vi "Main Scratch Module.vi"(8 "error in (no error)":errorcluster, 11 "main ref":T1) -> (0 "error out":errorcluster)   [LabVIEW 2025]
uses:
  controls/LAB-IQ UI Data.ctl
  Scratch Main Enum.ctl
  HEAVE vi's/Heave Write enum.ctl
  b016255a-5e45-488d-a19e-9ca17f1d2554.vi
  230b88c4-d326-49ea-ab42-a573b91a982d.vi
  e59e0919-8fad-4c7c-b2ce-8f9a2e4ae2bd.vi
panel:
  out "Scratch Start Recording":bool
  out "Multi Pass Count":dbl
  out "Multi Scratch with offset":bool
  out "Distance Moved unload":dbl
  out "PID Unload Temp":bool
  out "Scratch Backward Temp":bool
  out "Distance Moved Backward":dbl
  out "Distance Moved":dbl
  out "Scratch Forward Temp":bool
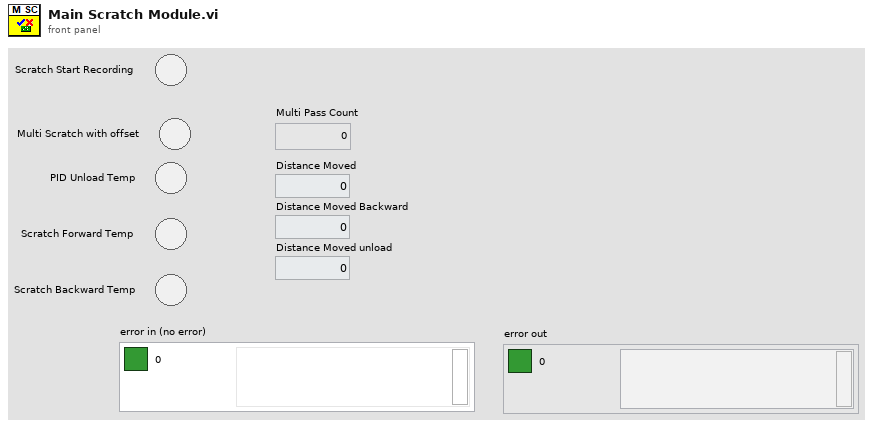
[diagram p1: front panel]
types:
  T1 = typedef "LAB-IQ UI Data.ctl" = cluster{"Main Home Screen":cluster{"GUI":refnum<vi>, "Platform Settings":refnum<vi>, "Configure":refnum<vi>, "Home":refnum<vi>, "EXIT":refnum<vi>, "service 2":refnum<vi>, "MainPage":refnum<vi>, "Analysis":refnum<vi>}, "Platform Settings":cluster{"mm/s  Surge":refnum<vi>, "Update Surge Speed":refnum<vi>, "Drive Error":refnum<vi>, "Disable Axis Jog Soft Limits":refnum<vi>, "mm/s  Sway":refnum<vi>, "Sway and Surge COM Status":refnum<vi>, "Heave COM Status":refnum<vi>, "Enable Platform":refnum<vi>, "Surge Forward Main":refnum<vi>, "Sway Right Main":refnum<vi>, "Sway Left Main":refnum<vi>, "Heave Down Main":refnum<vi>, "Heave Up main":refnum<vi>, "Update Sway Speed":refnum<vi>, "Update Heave Speed":refnum<vi>, "mm/s Heave":refnum<vi>, "mm/sec":refnum<vi>, "mm":refnum<vi>, "Surge Backward Main":refnum<vi>}, "Analysis Screen":cluster{"Analysis Home":refnum<vi>, "Surface Analysis":refnum<vi>, "Imaging":refnum<vi>, "Image Analysis":refnum<vi>, "Post Analysis":refnum<vi>}, "Config Screen":cluster{"Select Load Head":refnum<vi>, "Notes :":refnum<vi>, "FILE":refnum<vi>, "Sample ID :":refnum<vi>, "Operator ID :":refnum<vi>, "Operator Name :":refnum<vi>, "Auto":refnum<vi>}, "Motion Module":cluster{"zNL":refnum<vi>, "NL disp":refnum<vi>, "Rotary Tab":refnum<vi>, "Motion Direction:  3":refnum<vi>, "E.Velocity 2":refnum<vi>, "e.v/ssr 2":refnum<vi>, "Enter Fixed E.Velocity 2":refnum<vi>, "Enter Final SRR 2":refnum<vi>, "Enter initial SRR 2":refnum<vi>, "Enter Fixed SRR 2":refnum<vi>, "Enter the Final E.Velocity (m/s) 2":refnum<vi>, "Enter initial E.Velocity (m/s) 2":refnum<vi>, "Final Speed (RPM) 3":refnum<vi>, "Initial Speed (RPM) 2":refnum<vi>, "Enter the Final Velocity (m/s) 3":refnum<vi>, "Enter initial Velocity (m/s)  3":refnum<vi>, "Ramp Up 2":refnum<vi>, "TEST SELECTION":refnum<vi>, "SPEED SELECTION : ":refnum<vi>, "Angular Oscillation Set":refnum<vi>, "Traction":refnum<vi>, "Step Speed":refnum<vi>, "StepTable For Load-Speed":refnum<vi>, "StepTable For Speed":refnum<vi>, "Surge Forward MM":refnum<vi>, "Surge Backward MM":refnum<vi>, "M3 Image":refnum<vi>, "String 39":refnum<vi>, "Sway Left MM":refnum<vi>, "Sway Right MM":refnum<vi>, "Disable Axis Jog Soft Limits":refnum<vi>, "mm":refnum<vi>, "Heave Down MM":refnum<vi>, "Heave Up MM":refnum<vi>, "Wear Track Diameter (mm)":refnum<vi>, "Set WTD":refnum<vi>, "HomeScratch":refnum<vi>, "HomeRot":refnum<vi>, "PlaceModule":refnum<vi>, "Enter the Angle (Deg)":refnum<vi>, "Enter the Frequency (Hz)":refnum<vi>, "Motion Mode:":refnum<vi>, "LR Sway":refnum<vi>, "Rot Hor":refnum<vi>, "Scratch":refnum<vi>, "LR Cam":refnum<vi>, "MMBack":refnum<vi>, "MMNext":refnum<vi>, "Rot Ver":refnum<vi>, "Rotary Module Selection":refnum<vi>, "calculate rotary":refnum<vi>, "SPEED SELECTION : rotary":refnum<vi>, "Import 2":refnum<vi>, "Save 2":refnum<vi>, "File Path :  2":refnum<vi>, "String 45":refnum<vi>, "StepTable For Speed 3":refnum<vi>, "Enter the Speed(mm/sec)":refnum<vi>, "Enter the Speed(RPM)":refnum<vi>, "Enter Scratch Speed (mm/s):":refnum<vi>, "SwaySpeed Set":refnum<vi>, "Scartch Offset":refnum<vi>, "Motion type:":refnum<vi>, "HomeScratch 2":refnum<vi>, "Enter Scratch length (mm):":refnum<vi>, "Wear Track Diameter":refnum<vi>, "Rotary Speed Exced":refnum<vi>, "Scratch Mode":refnum<vi>, "No of Scratch":refnum<vi>}, "Environmental control":cluster{"Humidity  Status  3":refnum<vi>, "Low Temp  Status  2":refnum<vi>, "TK4 status 2":refnum<vi>, "Stage Temperature":refnum<vi>, "Sample Temperature":refnum<vi>, "Humidity (Amb)":refnum<vi>, "Clear List":refnum<vi>, "Add to list":refnum<vi>, "Wear":refnum<vi>, "Vibration":refnum<vi>, "Humidity (Chamber)":refnum<vi>, "Temperature (Chamber)":refnum<vi>, "ECR ":refnum<vi>, "Temperature (Amb)":refnum<vi>, "Microphone":refnum<vi>, "Acoustic Emission 3":refnum<vi>, "SNext":refnum<vi>, "APBack":refnum<vi>, "Enter the Temperature (°C):":refnum<vi>, "Enter the Stage \nTemperature (°C):":refnum<vi>, "Enter the Humidity (%Rh):":refnum<vi>, "Low Temp":refnum<vi>, "High Temp":refnum<vi>, "Humidity":refnum<vi>, "Sensors Picked":refnum<vi>}, "About Screen":cluster{"Password":refnum<vi>, "Home Service":refnum<vi>, "Advanced Setting":refnum<vi>, "About Tab":refnum<vi>, "ECR Port:":refnum<vi>, "Ramp Port:":refnum<vi>, "Installation/Replacement completed":refnum<vi>, "Loahead":refnum<vi>, "Heave and Surge COM Port:":refnum<vi>, "Sway COM Port:":refnum<vi>, "Temp Modbus:":refnum<vi>, "Humidity Port:":refnum<vi>, "Edit Gain Constants":refnum<vi>, "Save Gain Constants":refnum<vi>}, "Main Screen":cluster{"Main Screen Tab":refnum<vi>, "Angle and Frequency":refnum<vi>, "Stroke (mm)":refnum<vi>, "Angle (Deg)":refnum<vi>, "Main Speed Tab":refnum<vi>, "MTM MOTOR DISPLAY":refnum<vi>, "Disc Speed (m/sec)":refnum<vi>, "Ball Speed (m/sec)":refnum<vi>, "Disc Speed (RPM)":refnum<vi>, "Ball Speed (RPM)":refnum<vi>, "SPEED TAB":refnum<vi>, "Speed (m/sec)":refnum<vi>, "Set Speed (m/sec)":refnum<vi>, "Speed (RPM)":refnum<vi>, "Set Speed":refnum<vi>, "Time Tab":refnum<vi>, "Time ( HH:MM:SS ) 2":refnum<vi>, "Test Duration":refnum<vi>, "Test Duration 4":refnum<vi>, "TEST CYCLE":refnum<vi>, "TOTAL CYCLES":refnum<vi>, "Set Load (N)":refnum<vi>, "Temp Tabs":refnum<vi>, "Heater":refnum<vi>, "TK4 status":refnum<vi>, "ChamberTemp":refnum<vi>, "SetTmp":refnum<vi>, "Controller  Status":refnum<vi>, "ChamberTemp 2":refnum<vi>, "SetTmp 2":refnum<vi>, "Controller  Status 2":refnum<vi>, "ChamberTemp 3":refnum<vi>, "SetTmp 3":refnum<vi>, "Cooling":refnum<vi>, "Load Communication":refnum<vi>, "Ambient \nTemperature":refnum<vi>, "HumCOMStatus":refnum<vi>, "Ambient\n Humidity":refnum<vi>, "Freq (Hz)":refnum<vi>, "Load En":refnum<vi>, "NLt":refnum<vi>, "zNL 2":refnum<vi>, "Humidity On":refnum<vi>, "humidity disp":refnum<vi>, "Set Humidity":refnum<vi>, "NL disp 2":refnum<vi>, "Humidity On 2":refnum<vi>, "humidity disp 2":refnum<vi>, "Set Humidity 2":refnum<vi>, "NL disp 3":refnum<vi>, "AppLoadSeq scratch":refnum<vi>, "Stop Scratch":refnum<vi>, "ClrLog":refnum<vi>, "Trip Log":refnum<vi>, "STOP":refnum<vi>, "Start Test":refnum<vi>, "Test status":refnum<vi>, "AR Led":refnum<vi>, "Data":refnum<vi>, "Health":refnum<vi>, "Sway COM Status":refnum<vi>, "Heave COM Status":refnum<vi>, "Grp Tab":refnum<vi>, "Sub Graph":refnum<vi>, "SD (mm)":refnum<vi>, "Siliding distance Reset Graph":refnum<vi>, "SDGp":refnum<vi>, "Humidity Reset Graph":refnum<vi>, "HumrGp":refnum<vi>, "Acoustic Emission (mV)":refnum<vi>, "Aqucostic Reset Graph":refnum<vi>, "gACQUOS":refnum<vi>, "ECR RESET":refnum<vi>, "ECR":refnum<vi>, "Temperature Reset":refnum<vi>, "Acoustic Emission (mV) 2":refnum<vi>, "Aqucostic Reset Graph 2":refnum<vi>, "gACQUOS 2":refnum<vi>, "ECR RESET 2":refnum<vi>, "ECR 2":refnum<vi>, "Temperature Reset 2":refnum<vi>, "Temperature (deg c)":refnum<vi>, "Speed Reset Graph":refnum<vi>, "Speed Tab":refnum<vi>, "MTM DISC  SPEED":refnum<vi>, "MTM BALL SPEED":refnum<vi>, "speed mm/sec":refnum<vi>, "Hymidity":refnum<vi>, "Humidity Disable trip":refnum<vi>, "CoF Trip  2":refnum<vi>, "Depth Trip":refnum<vi>, "Weart Deapth":refnum<vi>, "Depth Reset Graph":refnum<vi>, "Weart":refnum<vi>, "Depthz":refnum<vi>, "Depth (µm)":refnum<vi>, "WearGp":refnum<vi>, "NL Trip 2":refnum<vi>, "Load pid":refnum<vi>, "Load Disable Trip":refnum<vi>, "Load Reset Graph":refnum<vi>, "NL Display 4":refnum<vi>, "Main Chart 3":refnum<vi>, "BACK":refnum<vi>, "Depth Trip 2":refnum<vi>, "COF TRIP ":refnum<vi>, "Friction Force (N)":refnum<vi>, "FF Reset Graph":refnum<vi>, "FF Disable Trip":refnum<vi>, "FF TRIP":refnum<vi>, "COF Disable Trip":refnum<vi>, "COF Reset Graph":refnum<vi>, "Start Test Temp":refnum<vi>, "zFF":refnum<vi>, "Friction Force (N) Graph":refnum<vi>, "Coefficient of Friction":refnum<vi>, "Scratch Start Test":refnum<vi>, "FF Tab":refnum<vi>, "Cyclic Friction Force (N)":refnum<vi>, "CZ FF":refnum<vi>, "Cyclic Friction Force (N) Graph":refnum<vi>, "Cyclic Coefficient of Friction":refnum<vi>, "Cyclic FF TRIP":refnum<vi>, "Cyclic FF Disable Trip":refnum<vi>, "cyclic COF Disable Trip":refnum<vi>, "cyclic COF TRIP":refnum<vi>, "cyclic COF Reset Graph":refnum<vi>, "Cyclic FF Reset Graph":refnum<vi>, "Test Trip":refnum<vi>, "Multi Scratch Pass":refnum<vi>}, "Loading":cluster{"Indentation":refnum<vi>, "Reference Sample":refnum<vi>, "Load Cell Communication Slide":refnum<vi>, "com 3":refnum<vi>, "com":refnum<vi>, "DecaForce COM Status":refnum<vi>, "Update":refnum<vi>, "Clear 3":refnum<vi>, "seq":refnum<vi>, "Stribeck table":refnum<vi>, "Stribeck Table  For loading":refnum<vi>, "Loading Mode":refnum<vi>, "Enter the Final Load (N)":refnum<vi>, "Enter the CoF Trip":refnum<vi>, "Enter the Friction Force Trip":refnum<vi>, "Enter the Normal load Trip":refnum<vi>, "Enter the Load  (N)":refnum<vi>, "KiloForce":refnum<vi>, "DecaForce ":refnum<vi>, "MicroForce":refnum<vi>, "LHBack":refnum<vi>, "LHNext":refnum<vi>, "Enter the Loading Rate (N/min)":refnum<vi>, "Message":refnum<vi>, "Warning 2":refnum<vi>, "SSP 0.75":refnum<vi>, "SSP 0.5":refnum<vi>, "SSP 0.3":refnum<vi>, "Warning":refnum<vi>, "gui GIF":refnum<vi>, "Communication is established":refnum<vi>, "AppLoad 4":refnum<vi>, "Multipoint":refnum<vi>, "Load Selection":refnum<vi>}, "PID":cluster{"Ramp MulFac":refnum<vi>, "pulses LoadDiffRamp(2..10)":refnum<vi>, "PulseControlRamp(diff<=3N)":refnum<vi>, "SetLoadDeadband(%) Load(0-10N)":refnum<vi>, "PID gains out delay (microForce)":refnum<vi>, "Ramp":refnum<vi>, "Gain 2":refnum<vi>, "pulses LoadDiff(2..10)":refnum<vi>, "pulses LoadDiff(11..50)":refnum<vi>, "PulseControl(diff<=3N)":refnum<vi>, "SetLoadDeadband(%)  2":refnum<vi>, "Dummy Run":refnum<vi>, "Vertical load (N)":refnum<vi>, "AutoTune":refnum<vi>, "Offset 3 ":refnum<vi>, "apply load":refnum<vi>, "Offset  3":refnum<vi>, "apply load 2":refnum<vi>, "Enter ByPass Load":refnum<vi>, "reinit 3":refnum<vi>, "output range delay":refnum<vi>, "PID gains out delay":refnum<vi>, "Bypass Load":refnum<vi>, "pulsesSent":refnum<vi>, "pulses ":refnum<vi>, "actpid":refnum<vi>, "gFF Rot":refnum<vi>, "pulses LoadDiff(21..1000)":refnum<vi>, "Delay":refnum<vi>, "deadband":refnum<vi>}, "Config Parameters":cluster{"Tab Control 3":refnum<vi>, "Tab Control 19":refnum<vi>, "SAMPLES":refnum<vi>, "Re-initilaize":refnum<vi>, "Filter ON/OFF":refnum<vi>, "TracHomeSurgeOffsetCounts 10MM":refnum<vi>, "TracHomeSwayOffsetCounts 10MM":refnum<vi>, "Acoustic Emission:":refnum<vi>, "Apply Filter (FF)":refnum<vi>, "Filter% 2":refnum<vi>, "Apply Filter (Load)":refnum<vi>, "Filter% ":refnum<vi>, "Sway distance (mm)":refnum<vi>, "Surge distance (mm)":refnum<vi>, "DataSavingLoopDelay(ms)":refnum<vi>, "SAVE 2":refnum<vi>, "Enter Distance":refnum<vi>, "Sway Counts:":refnum<vi>, "Distance (mm): 3":refnum<vi>, "Surge Counts:":refnum<vi>, "Distance (mm): 2":refnum<vi>, "Distance (mm):":refnum<vi>, "Heave Counts:":refnum<vi>, "LRMHomeSurgeOffsetCounts":refnum<vi>, "LRMHomeSwayOffsetCounts":refnum<vi>, "TracHomeSurgeOffsetCounts 20MM":refnum<vi>, "TracHomeSwayOffsetCounts 20MM":refnum<vi>, "RotHomeSwayOffsetCounts":refnum<vi>, "RotHomeSurgeOffsetCounts":refnum<vi>, "Heave distance":refnum<vi>, "Zmm":refnum<vi>, "Heave Pulses/mm":refnum<vi>, "Surge Pulses/mm":refnum<vi>, "Sway Pulses/mm":refnum<vi>, "Heave Pitch":refnum<vi>, "Surge Pitch":refnum<vi>, "Sway Pitch":refnum<vi>, "Heave PPR":refnum<vi>, "Surge PPR":refnum<vi>, "Sway PPR":refnum<vi>, "Tab Control 5":refnum<vi>, "Tab Control 14":refnum<vi>, "Tab Control 26":refnum<vi>, "AE":refnum<vi>, "Heave Loop Delay":refnum<vi>, "Heave PID Speed":refnum<vi>, "Surge Jog Speed":refnum<vi>, "Heave Jog Speed":refnum<vi>, "Sway Loop Delay":refnum<vi>, "Sway PID Speed":refnum<vi>, "Sway Jog Speed":refnum<vi>}, "Loading Com Port":cluster{"ClearAll":refnum<vi>, "Mz(Nm)":refnum<vi>, "My(Nm)":refnum<vi>, "Mx(Nm)":refnum<vi>, "Save Dwell":refnum<vi>, "Mx ":refnum<vi>, "My ":refnum<vi>, "Mz":refnum<vi>, "Fx(N)":refnum<vi>, "Fy(N)":refnum<vi>, "Fz(N)":refnum<vi>, "ZeroAll":refnum<vi>, "Acq Delay (ms)":refnum<vi>, "Burst Delay (ms)":refnum<vi>, "model":refnum<vi>, "SN":refnum<vi>, "FFx(N)":refnum<vi>, "Sensor IP":refnum<vi>, "Port":refnum<vi>, "FFy(N)":refnum<vi>, "Load(N)":refnum<vi>, "delete Handle":refnum<vi>, "Create Handle":refnum<vi>, "ft_data":refnum<vi>, "ft_range":refnum<vi>, "ft_data 2":refnum<vi>, "stop 6":refnum<vi>, "running_flag":refnum<vi>, "ft_udp_handle":refnum<vi>, "get-data-return":refnum<vi>, "get-range-return":refnum<vi>, "zero-return":refnum<vi>, "filter-return":refnum<vi>, "initial-return":refnum<vi>, "deleteHandle-result":refnum<vi>, "Load Cell Temp":refnum<vi>}, "Heave AND Surge":cluster{"SURGE POSE":refnum<vi>, "error out Read":refnum<vi>, "HEAVE POSE":refnum<vi>, "State":refnum<vi>, "Homed":refnum<vi>, "Sequence ID":refnum<vi>, "error out Write":refnum<vi>, "faultCode":refnum<vi>, "Ack ID":refnum<vi>, "SPEED":refnum<vi>, "Distance":refnum<vi>, "Mode Command":refnum<vi>, "Heave and Surge Read":refnum<vi>, "Read Heave Temp":refnum<vi>, "Spare 15":refnum<vi>, "Spare 14":refnum<vi>, "Spare 13":refnum<vi>, "Spare 12":refnum<vi>, "Spare 11":refnum<vi>, "Spare 10":refnum<vi>, "Spare 9":refnum<vi>, "Spare 8":refnum<vi>, "Spare 7":refnum<vi>, "Spare 6":refnum<vi>, "Spare 5":refnum<vi>, "Spare 4":refnum<vi>, "Spare 2":refnum<vi>, "Spare 1":refnum<vi>, "Node Id":refnum<vi>, "Spare 3":refnum<vi>, "SPARE 4":refnum<vi>, "SPARE 3":refnum<vi>, "SPARE 2":refnum<vi>, "SPARE 1":refnum<vi>, "fwMajor":refnum<vi>, "fwMinor":refnum<vi>, "Manual Write":refnum<vi>, "Heave and Surge Write":refnum<vi>}, "New PID LOGIC":cluster{"Fine Tune Zone":refnum<vi>, "PID SDelay":refnum<vi>, "Max_pos_limit":refnum<vi>, "Min_pos_limit":refnum<vi>, "i_limit":refnum<vi>, "pct_scale":refnum<vi>, "Deadband":refnum<vi>, "Kd":refnum<vi>, "Ki":refnum<vi>, "Kp":refnum<vi>, "Current Position":refnum<vi>, "Set Load":refnum<vi>, "Current Load":refnum<vi>, "Pulse delta":refnum<vi>, "Init Step":refnum<vi>, "Max Step Linit":refnum<vi>}, "SWAY ":cluster{"fwMajor":refnum<vi>, "Homed":refnum<vi>, "Rotary POSE":refnum<vi>, "State":refnum<vi>, "SWAY POSE":refnum<vi>, "Ack ID":refnum<vi>, "faultCode":refnum<vi>, "Node Id":refnum<vi>, "fwMinor":refnum<vi>, "Spare 6":refnum<vi>, "Spare 5":refnum<vi>, "Spare 4":refnum<vi>, "Spare 3":refnum<vi>, "Spare 2":refnum<vi>, "Spare 1":refnum<vi>, "Spare 7":refnum<vi>, "SPARE  5":refnum<vi>, "error out Write  SWAY ":refnum<vi>, "error out Read SWAY ":refnum<vi>, "Manual Write SWAY ":refnum<vi>, "SWAY WRITE":refnum<vi>, "SPARE  4":refnum<vi>, "SPARE  3":refnum<vi>, "SPARE 2":refnum<vi>, "SPARE 1":refnum<vi>, "Spare 15":refnum<vi>, "Spare 14":refnum<vi>, "Spare 13":refnum<vi>, "Spare 12":refnum<vi>, "Spare 11":refnum<vi>, "Spare 9":refnum<vi>, "Spare 8":refnum<vi>, "SPEED":refnum<vi>, "Distance":refnum<vi>, "Mode Command":refnum<vi>, "Sequence ID":refnum<vi>, "SWAY READ":refnum<vi>, "Spare 10":refnum<vi>, "Read SWAY Temp":refnum<vi>}, "Analysis Screen":cluster{"Analysis Home":refnum<vi>, "Refresh 2":refnum<vi>, "MEAN 4":refnum<vi>, "SD 4":refnum<vi>, "VARIANCE 4":refnum<vi>, "MEAN  3":refnum<vi>, "SD  3":refnum<vi>, "VARIANCE  3":refnum<vi>, "MEAN 2":refnum<vi>, "SD  2":refnum<vi>, "VARIANCE 2":refnum<vi>, "MEAN":refnum<vi>, "SD":refnum<vi>, "VARIANCE":refnum<vi>, "File 4 Discription":refnum<vi>, "OPEN 4":refnum<vi>, "File Name 4":refnum<vi>, "OPEN 3":refnum<vi>, "File 3 Discription":refnum<vi>, "File Name 3":refnum<vi>, "Y-AXIS":refnum<vi>, "X-AXIS":refnum<vi>, "XY Graph":refnum<vi>, "File Name 2":refnum<vi>, "File Name 1":refnum<vi>, "OPEN 2":refnum<vi>, "OPEN 1":refnum<vi>, "File 1 Discription ":refnum<vi>, "File 2 Discription":refnum<vi>}}
  T2 = enum32{"Setup", "Load Head", "Motion Module", "Environment", "Begin"}
  T3 = typedef "Scratch Main Enum.ctl" = enum16{"Init", "Start", "Load", "Scratch Forward", "Scratch Backward", "Unload", "Offest", "Close"}
  T4 = typedef "Heave Write enum.ctl" = enum16{"INIT", "WRITE", "CLOSE", "REINIT"}
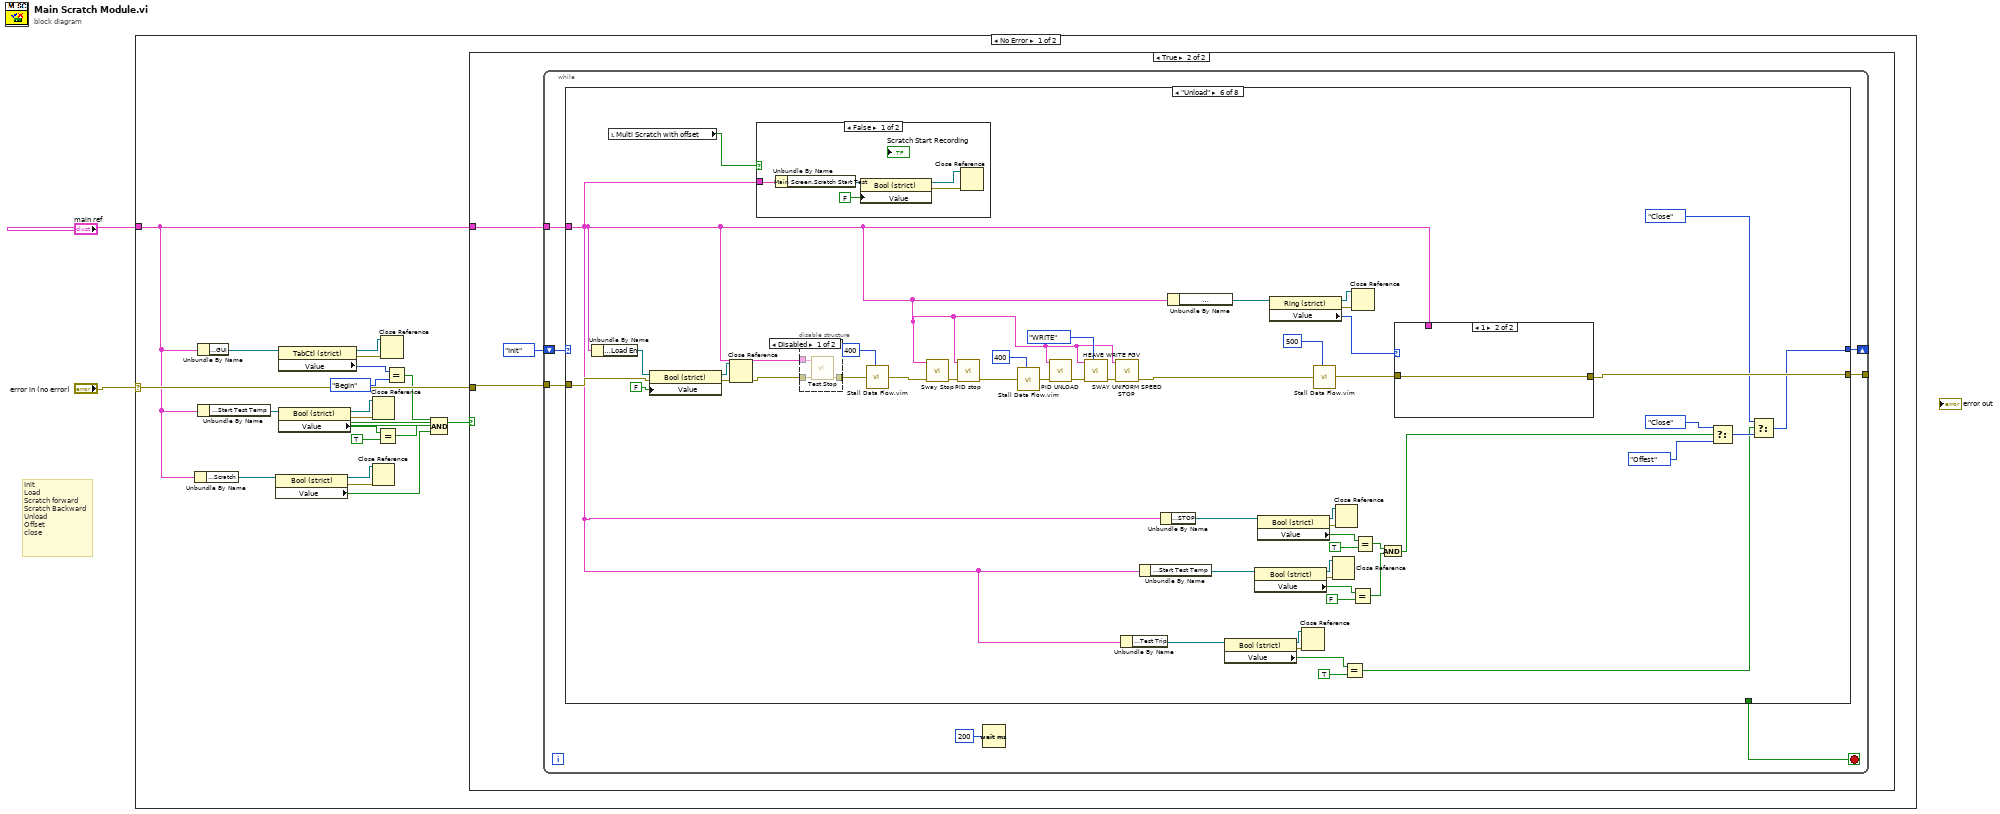
[diagram p0: block diagram]
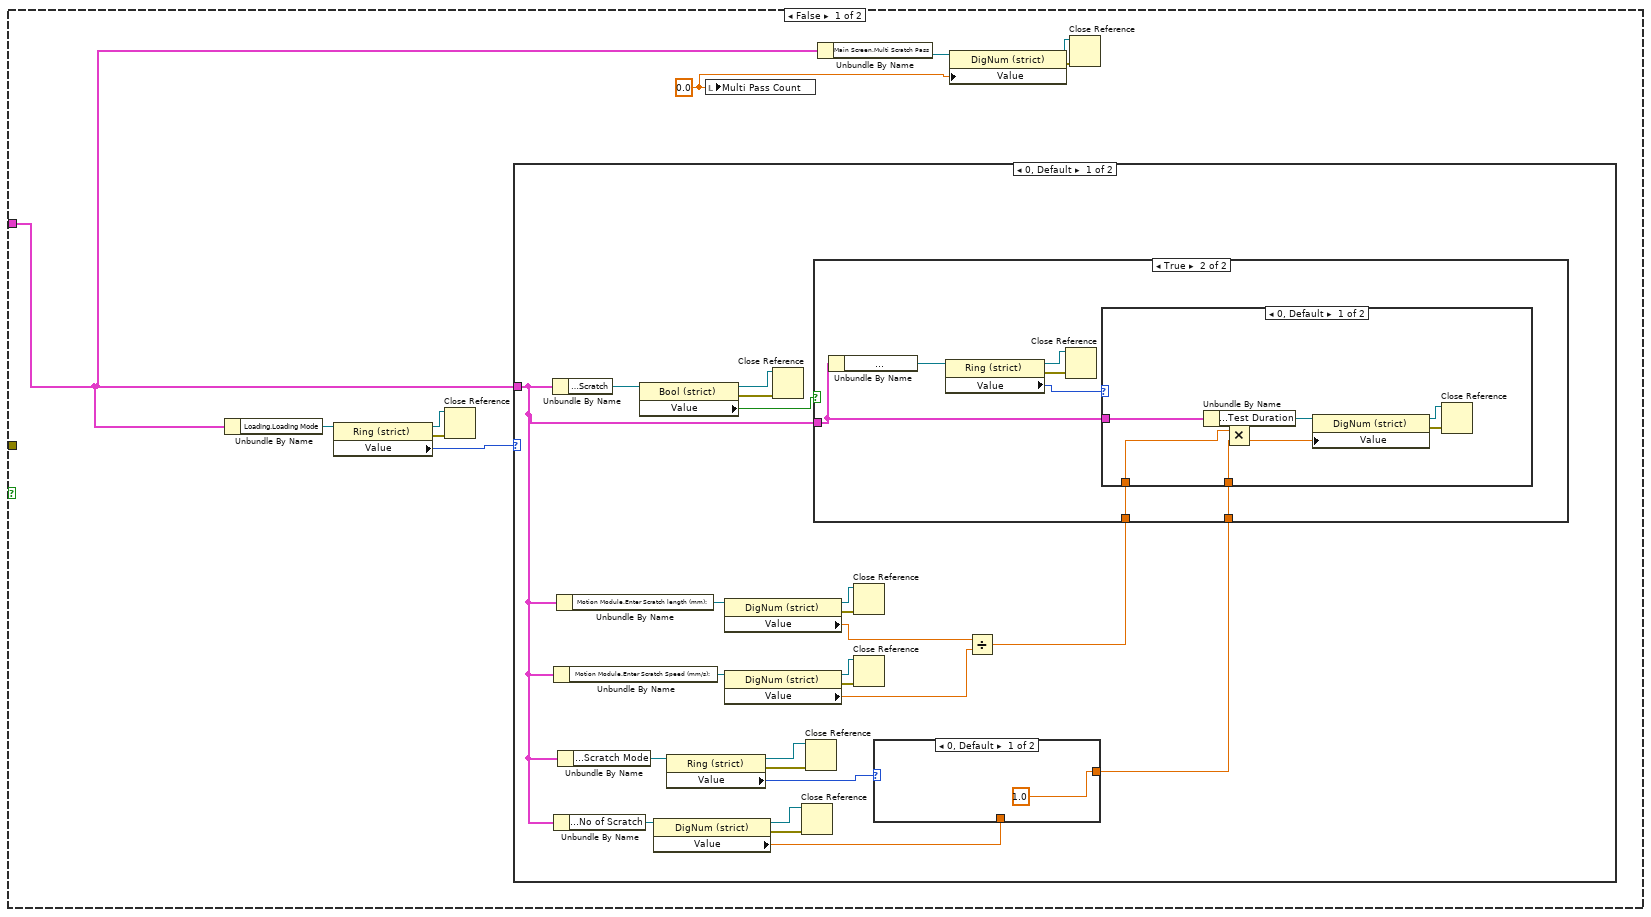
[diagram p2: hidden frame]
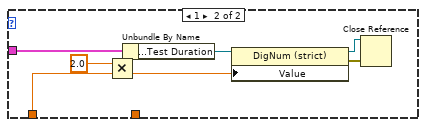
[diagram p5: hidden frame]
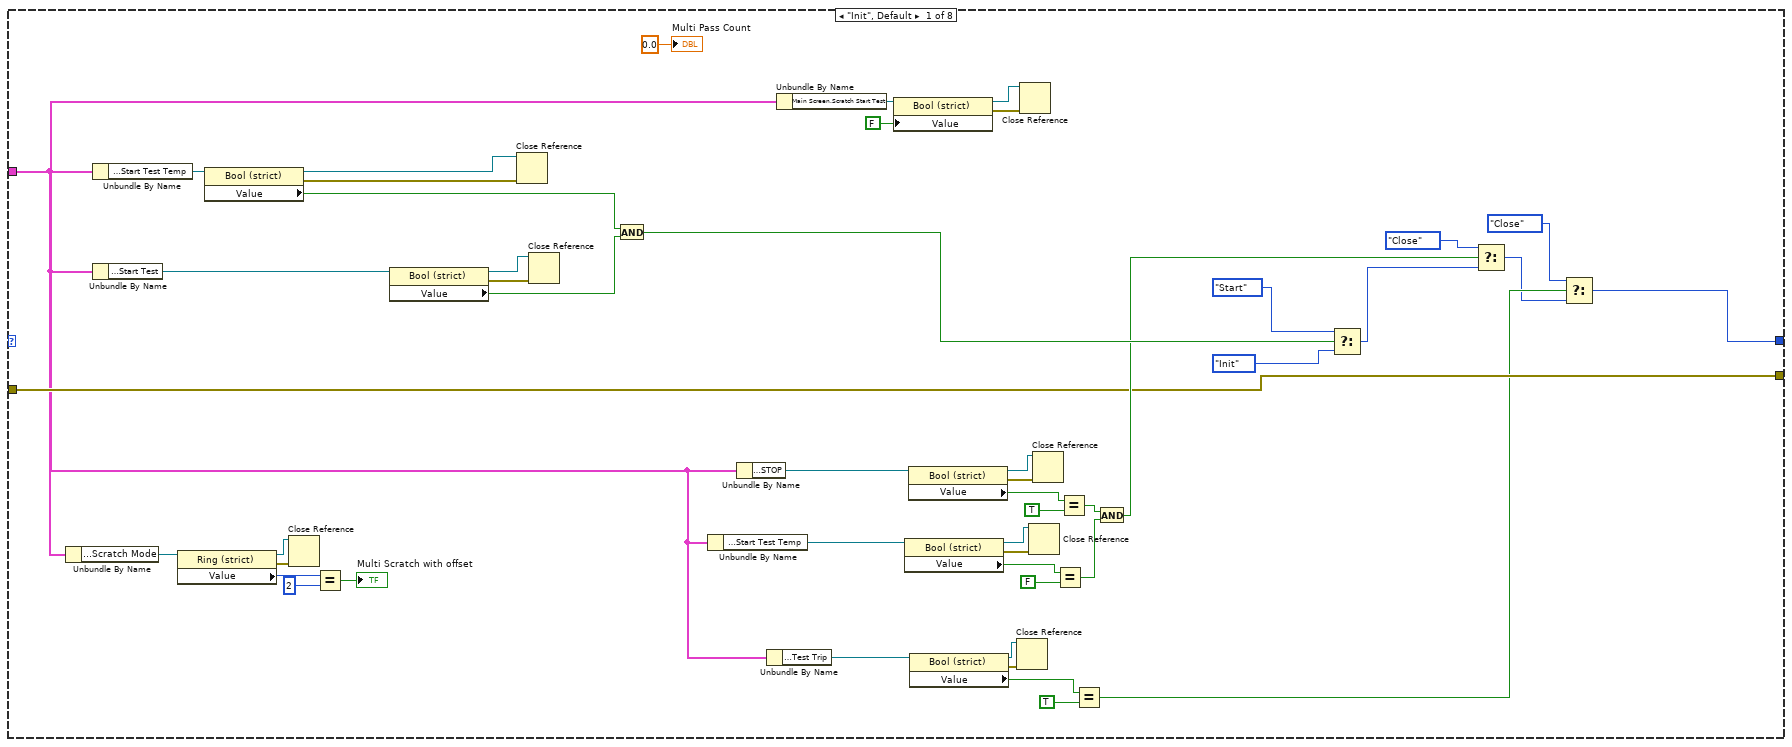
[diagram p7: hidden frame]
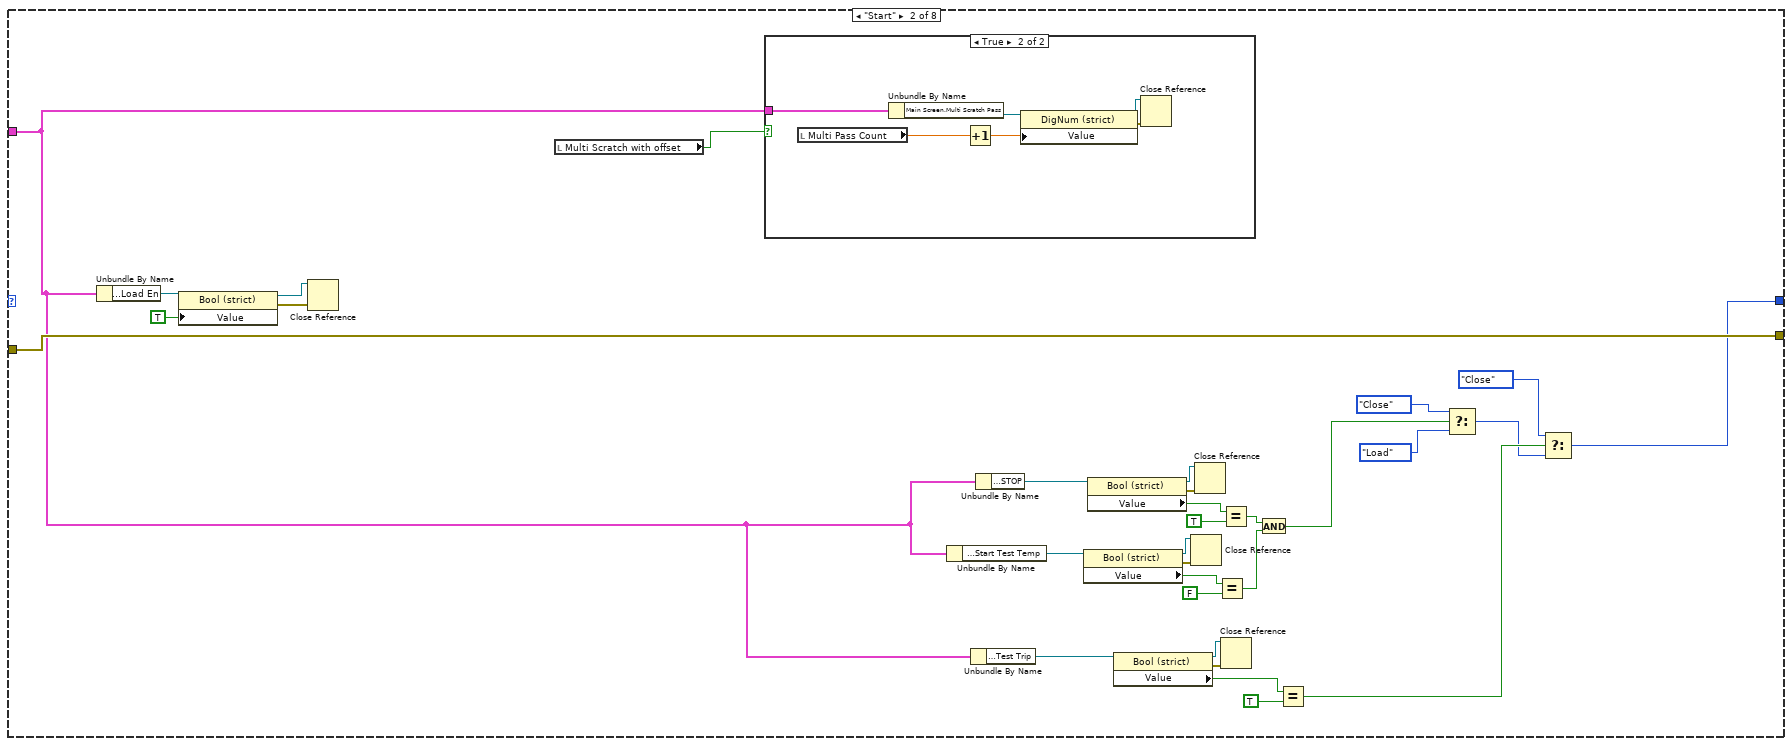
[diagram p8: hidden frame]
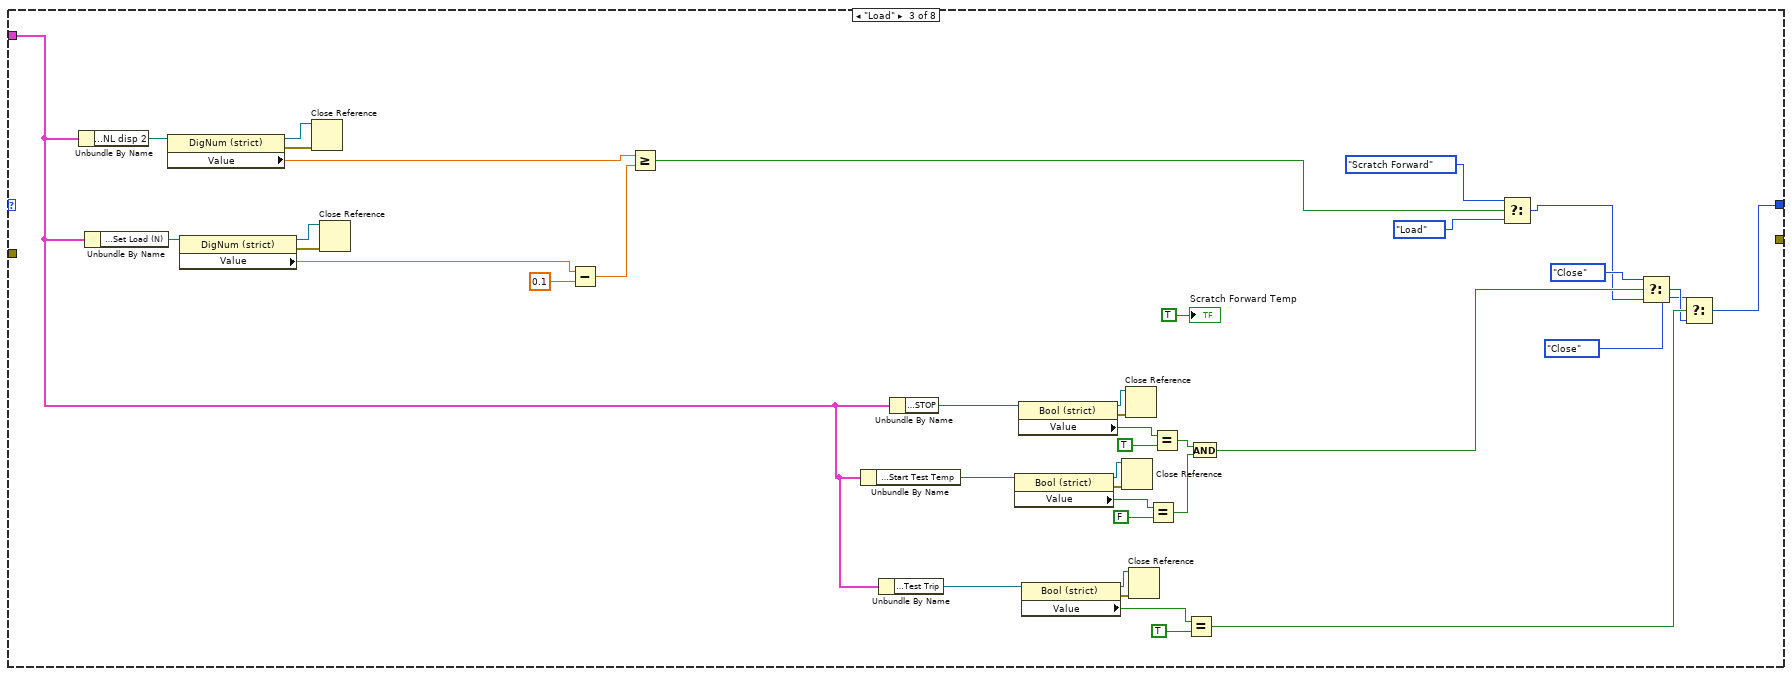
[diagram p10: hidden frame]
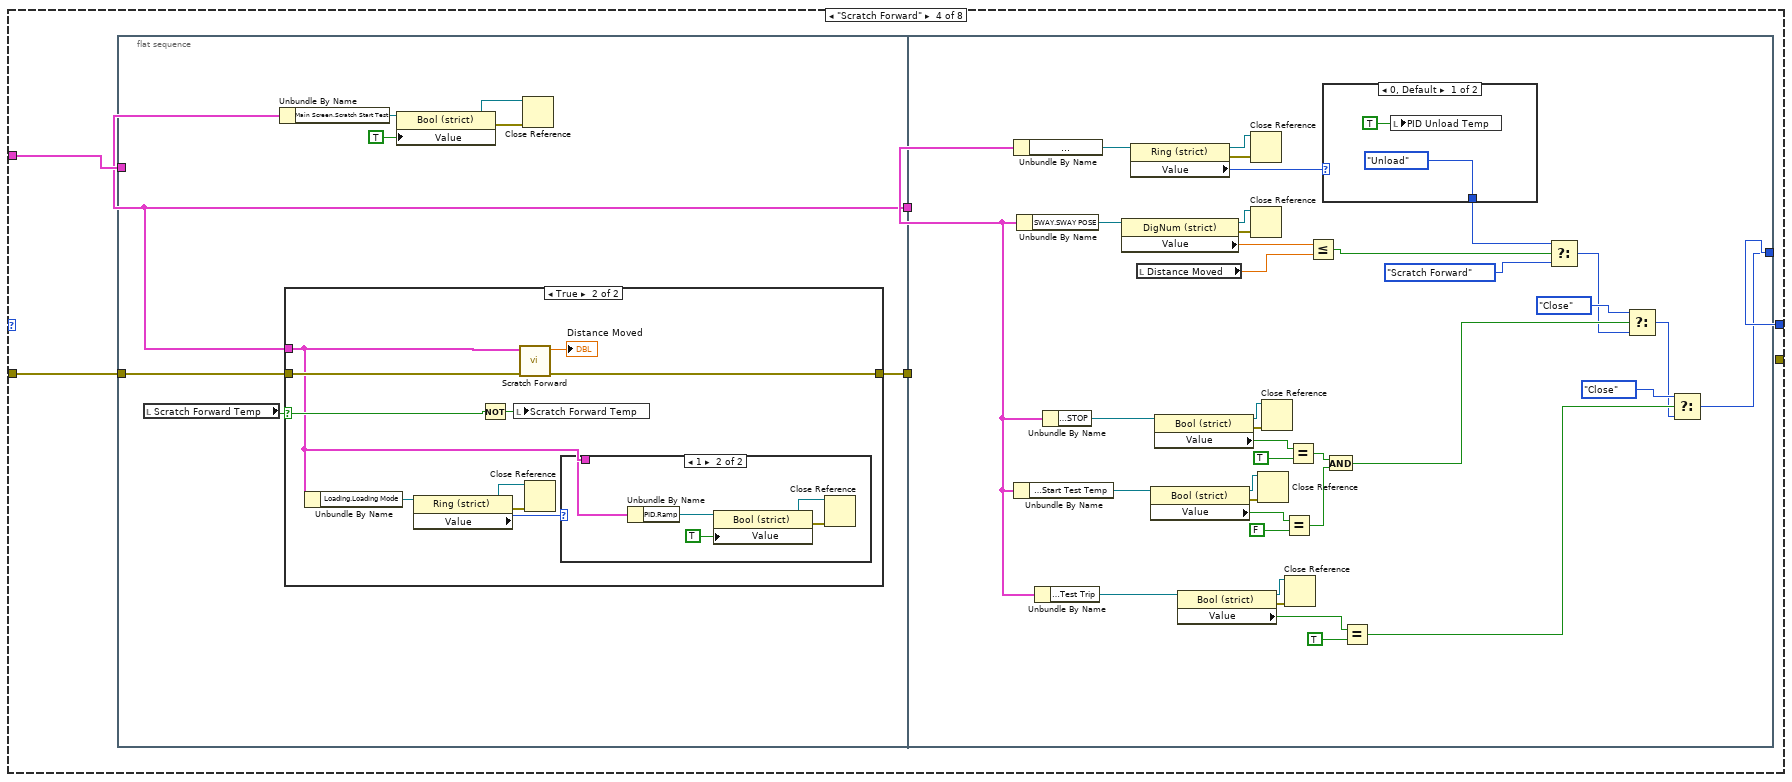
[diagram p11: hidden frame]
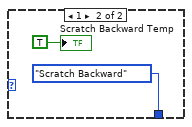
[diagram p14: hidden frame]
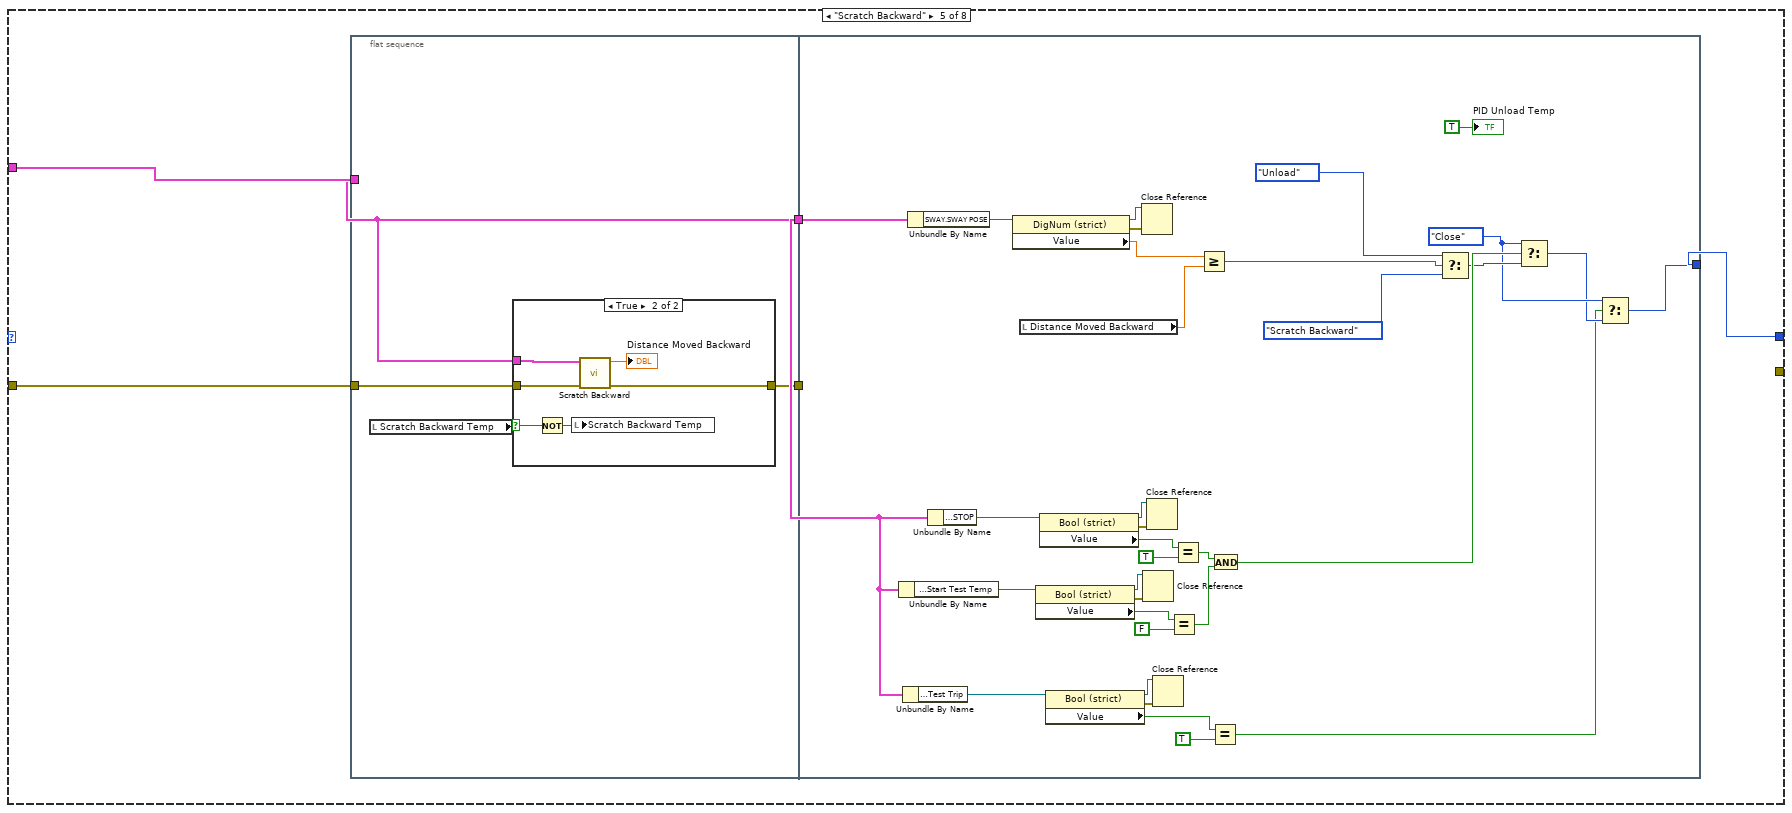
[diagram p15: hidden frame]
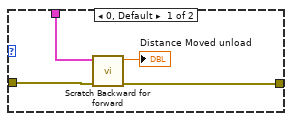
[diagram p19: hidden frame]
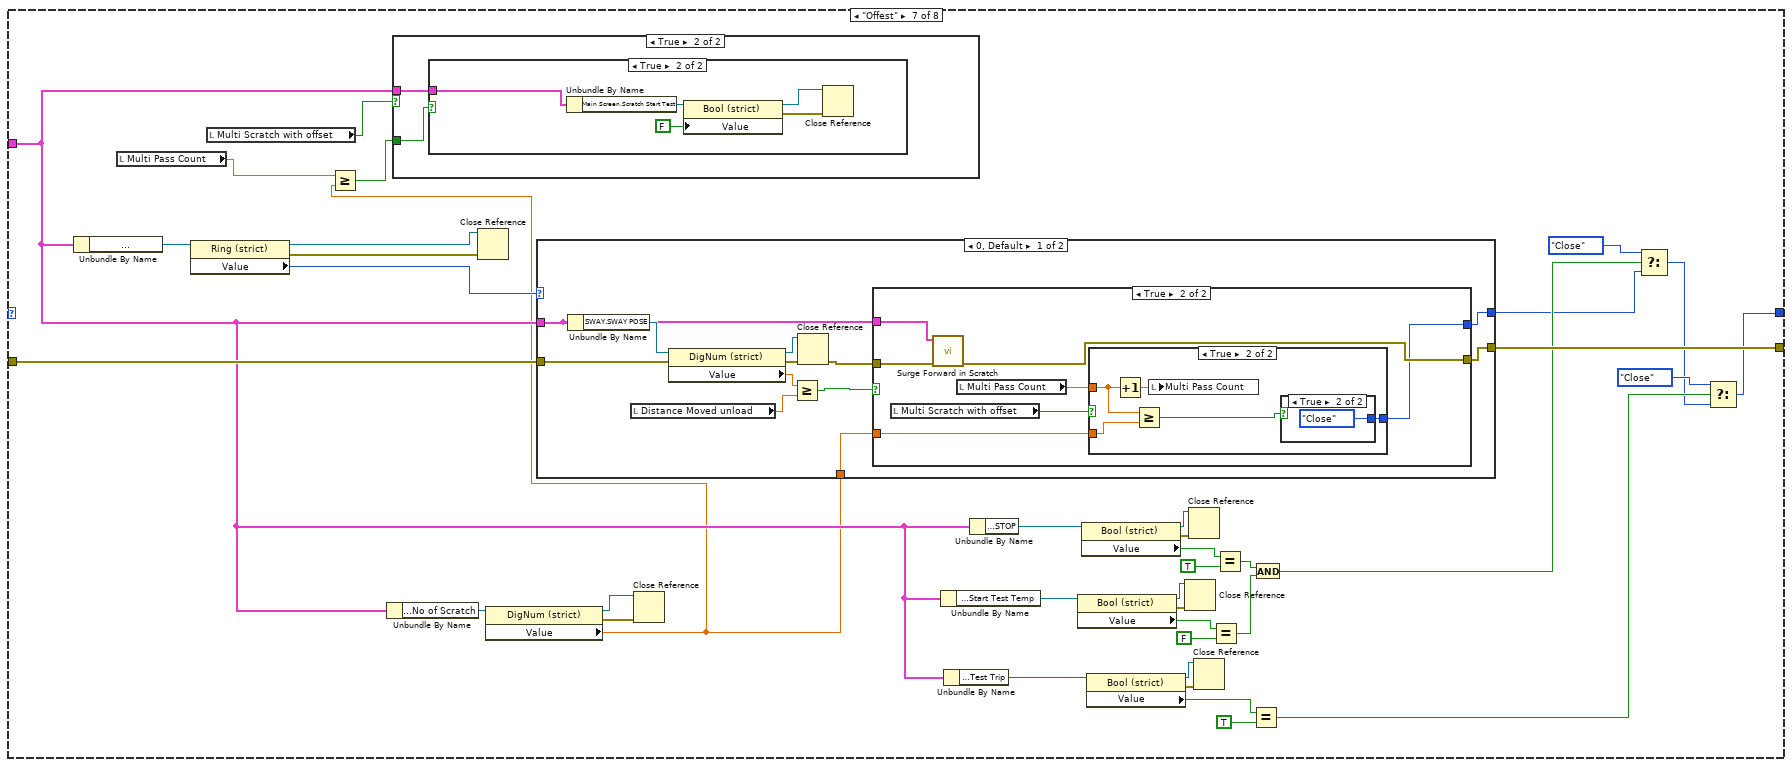
[diagram p20: hidden frame]
diagram:
  # "Init \nLoad\nScratch forward\nScratch Backward\nUnload\nOffset\nclose"
  n1 = case shown="No Error" "error in (no error)" {
    selector: "error in (no error)" -> [w21 _]
    tunnel: "main ref" -> [w4 _]
    frame No Error {
      n2 = Unbundle By Name(w4) -> ("Motion Module.Scratch"=w8:refnum<vi>)
      n3 = Unbundle By Name(w4) -> ("Main Home Screen.GUI"=w18:refnum<vi>)
      n4 = Unbundle By Name(w4) -> ("Main Screen.Start Test Temp"=w13:refnum<vi>)
      n5 = property class="Bool (strict)"(reference=w8) -> (reference out=w5:refnum<vi>, error out=w7:errorcluster, "Value"=w6:bool)  [unwired: 1 in]
      n6 = property class="TabCtl (strict)"(reference=w18) -> (reference out=w20:refnum<vi>, error out=w19:errorcluster, "Value"=w17:T2)  [unwired: 1 in]
      n7 = property class="Bool (strict)"(reference=w13) -> (reference out=w11:refnum<vi>, error out=w12:errorcluster, "Value"=w14:bool)  [unwired: 1 in]
      n8 = Close Reference(reference=w11, error in (no error)=w12) -> ()  [unwired: 1 out]
      n9 = Close Reference(reference=w5, error in (no error)=w7) -> ()  [unwired: 1 out]
      n10 = Equal?(x=w14, y=TRUE) -> (x = y?=w10:bool)
      n11 = Close Reference(reference=w20, error in (no error)=w19) -> ()  [unwired: 1 out]
      n12 = Equal?(x=w17, y=T2."Begin" ("Value")) -> (x = y?=w15:bool)
      n13 = Compound Arithmetic op=AND(w15, w10, w6) -> (w3:bool)
      n14 = case shown="True" w3 {
        tunnel: w4 -> [w23 w78]
        tunnel: w21 -> [_ w77]
        frame False {
          w22 = 0.0 ("Multi Pass Count")
          n15 = Unbundle By Name(w23) -> ("Loading.Loading Mode"=w30:refnum<vi>)
          n16 = property class="Ring (strict)"(reference=w30) -> (reference out=w28:refnum<vi>, error out=w29:errorcluster, "Value"=w27:u16)  [unwired: 1 in]
          n17 = Close Reference(reference=w28, error in (no error)=w29) -> ()  [unwired: 1 out]
          n18 = case shown="0, Default" w27 {
            tunnel: w23 -> [w33 _]
            frame 0, Default {
              n19 = Unbundle By Name(w33) -> ("Motion Module.Scratch"=w51:refnum<vi>)
              n20 = Unbundle By Name(w33) -> ("Motion Module.Enter Scratch Speed (mm/s):"=w46:refnum<vi>)
              n21 = Unbundle By Name(w33) -> ("Motion Module.No of Scratch"=w35:refnum<vi>)
              n22 = Unbundle By Name(w33) -> ("Motion Module.Enter Scratch length (mm):"=w47:refnum<vi>)
              n23 = Unbundle By Name(w33) -> ("Motion Module.Scratch Mode"=w39:refnum<vi>)
              n24 = property class="Bool (strict)"(reference=w51) -> (reference out=w53:refnum<vi>, error out=w52:errorcluster, "Value"=w50:bool)  [unwired: 1 in]
              n25 = property class="DigNum (strict)"(reference=w35) -> (reference out=w34:refnum<vi>, error out=w36:errorcluster, "Value"=w32:dbl)  [unwired: 1 in]
              n26 = property class="Ring (strict)"(reference=w39) -> (reference out=w40:refnum<vi>, error out=w38:errorcluster, "Value"=w37:u16)  [unwired: 1 in]
              n27 = property class="DigNum (strict)"(reference=w47) -> (reference out=w49:refnum<vi>, error out=w48:errorcluster, "Value"=w43:dbl)  [unwired: 1 in]
              n28 = property class="DigNum (strict)"(reference=w46) -> (reference out=w44:refnum<vi>, error out=w45:errorcluster, "Value"=w42:dbl)  [unwired: 1 in]
              n29 = Close Reference(reference=w53, error in (no error)=w52) -> ()  [unwired: 1 out]
              n30 = Close Reference(reference=w34, error in (no error)=w36) -> ()  [unwired: 1 out]
              n31 = Close Reference(reference=w40, error in (no error)=w38) -> ()  [unwired: 1 out]
              n32 = Close Reference(reference=w49, error in (no error)=w48) -> ()  [unwired: 1 out]
              n33 = Close Reference(reference=w44, error in (no error)=w45) -> ()  [unwired: 1 out]
              n34 = case shown="0, Default" w37 {
                tunnel: [1.0 w55] -> w31
                tunnel: w32 -> [_ w55]
                frame 0, Default {
                }
                frame 2 {
                }
              }
              n35 = Divide(x=w43, y=w42) -> (x/y=w41:dbl)
              n36 = case shown="True" w50 {
                tunnel: w33 -> [_ w57]
                tunnel: w41 -> [_ w58]
                tunnel: w31 -> [_ w56]
                frame False {
                }
                frame True {
                  n37 = Unbundle By Name(w57) -> ("Motion Module.Motion type:"=w61:refnum<vi>)
                  n38 = property class="Ring (strict)"(reference=w61) -> (reference out=w62:refnum<vi>, error out=w60:errorcluster, "Value"=w59:u16)  [unwired: 1 in]
                  n39 = Close Reference(reference=w62, error in (no error)=w60) -> ()  [unwired: 1 out]
                  n40 = case shown="0, Default" w59 {
                    tunnel: w58 -> [w64 w72]
                    tunnel: w57 -> [w66 w73]
                    tunnel: w56 -> [w63 _]
                    frame 0, Default {
                      n41 = Unbundle By Name(w66) -> ("Main Screen.Test Duration"=w68:refnum<vi>)
                      n42 = Multiply(x=w64, y=w63) -> (x*y=w65:dbl)
                      n43 = property class="DigNum (strict)"(reference=w68, "Value"=w65) -> (reference out=w69:refnum<vi>, error out=w67:errorcluster)  [unwired: 1 in]
                      n44 = Close Reference(reference=w69, error in (no error)=w67) -> ()  [unwired: 1 out]
                    }
                    frame 1 {
                      n45 = Multiply(x=2.0, y=w72) -> (x*y=w71:dbl)
                      n46 = Unbundle By Name(w73) -> ("Main Screen.Test Duration"=w75:refnum<vi>)
                      n47 = property class="DigNum (strict)"(reference=w75, "Value"=w71) -> (reference out=w76:refnum<vi>, error out=w74:errorcluster)  [unwired: 1 in]
                      n48 = Close Reference(reference=w76, error in (no error)=w74) -> ()  [unwired: 1 out]
                    }
                  }
                }
              }
            }
            frame 1 {
            }
          }
          n49 = local write "Multi Pass Count"(w22) -> ()
          n50 = Unbundle By Name(w23) -> ("Main Screen.Multi Scratch Pass"=w26:refnum<vi>)
          n51 = property class="DigNum (strict)"(reference=w26, "Value"=w22) -> (reference out=w24:refnum<vi>, error out=w25:errorcluster)  [unwired: 1 in]
          n52 = Close Reference(reference=w24, error in (no error)=w25) -> ()  [unwired: 1 out]
        }
        frame True {
          n53 = while {
            shift-right: [w84] -> _
            shift-left: Scratch_Main_Enum."Init" -> [w86]
            tunnel: w78 -> [w85]
            tunnel: w77 -> [w83]
            tunnel: [w81] -> _
            stop <- w80 stop-if-true
            n54 = case shown="\"Unload\"" w86 {
              tunnel: w85 -> [w89 w135 w176 w215 w285 w337 w398 w479]
              tunnel: [w95 w137 w172 w211 w281 w331 w402 Scratch_Main_Enum."Init"] -> w84
              tunnel: w83 -> [w108 w161 _ w214 w284 w343 w431 w487]
              tunnel: [w108 w161 _ _ _ w375 w426 w485] -> w81
              tunnel: [_ _ _ _ _ _ _ TRUE] -> w80
              frame "Init", Default {
                n55 = Unbundle By Name(w89) -> ("Motion Module.Scratch Mode"=w93:refnum<vi>)
                n56 = Unbundle By Name(w89) -> ("Main Screen.Start Test Temp"=w131:refnum<vi>)
                n57 = Unbundle By Name(w89) -> ("Main Screen.Start Test"=w128:refnum<vi>)
                n58 = property class="Ring (strict)"(reference=w93) -> (reference out=w94:refnum<vi>, error out=w92:errorcluster, "Value"=w91:u16)  [unwired: 1 in]
                n59 = property class="Bool (strict)"(reference=w131) -> (reference out=w132:refnum<vi>, error out=w130:errorcluster, "Value"=w126:bool)  [unwired: 1 in]
                n60 = Close Reference(reference=w94, error in (no error)=w92) -> ()  [unwired: 1 out]
                n61 = Equal?(x=w91, y=u16 2) -> (x = y?=→"Multi Scratch with offset":bool)
                n62 = property class="Bool (strict)"(reference=w128) -> (reference out=w127:refnum<vi>, error out=w129:errorcluster, "Value"=w125:bool)  [unwired: 1 in]
                n63 = Close Reference(reference=w132, error in (no error)=w130) -> ()  [unwired: 1 out]
                n64 = Close Reference(reference=w127, error in (no error)=w129) -> ()  [unwired: 1 out]
                n65 = And(x=w126, y=w125) -> (x .and. y?=w124:bool)
                n66 = Unbundle By Name(w89) -> ("Main Screen.Start Test Temp"=w118:refnum<vi>)
                n67 = Unbundle By Name(w89) -> ("Main Screen.STOP"=w121:refnum<vi>)
                n68 = Unbundle By Name(w89) -> ("Main Screen.Test Trip"=w101:refnum<vi>)
                n69 = Unbundle By Name(w89) -> ("Main Screen.Scratch Start Test"=w106:refnum<vi>)
                n70 = property class="Bool (strict)"(reference=w106, "Value"=FALSE) -> (reference out=w107:refnum<vi>, error out=w105:errorcluster)  [unwired: 1 in]
                n71 = property class="Bool (strict)"(reference=w118) -> (reference out=w116:refnum<vi>, error out=w117:errorcluster, "Value"=w119:bool)  [unwired: 1 in]
                n72 = property class="Bool (strict)"(reference=w121) -> (reference out=w123:refnum<vi>, error out=w122:errorcluster, "Value"=w120:bool)  [unwired: 1 in]
                n73 = property class="Bool (strict)"(reference=w101) -> (reference out=w103:refnum<vi>, error out=w102:errorcluster, "Value"=w99:bool)  [unwired: 1 in]
                n74 = Close Reference(reference=w103, error in (no error)=w102) -> ()  [unwired: 1 out]
                n75 = Close Reference(reference=w107, error in (no error)=w105) -> ()  [unwired: 1 out]
                n76 = Close Reference(reference=w116, error in (no error)=w117) -> ()  [unwired: 1 out]
                n77 = Close Reference(reference=w123, error in (no error)=w122) -> ()  [unwired: 1 out]
                n78 = Equal?(x=w119, y=FALSE) -> (x = y?=w114:bool)
                n79 = Equal?(x=w120, y=TRUE) -> (x = y?=w115:bool)
                n80 = Equal?(x=w99, y=TRUE) -> (x = y?=w98:bool)
                n81 = And(x=w115, y=w114) -> (x .and. y?=w111:bool)
                n82 = Select(t=Scratch_Main_Enum."Start", s=w124, f=Scratch_Main_Enum."Init") -> (s? t:f=w109:T3)
                n83 = Select(t=Scratch_Main_Enum."Close", s=w111, f=w109) -> (s? t:f=w96:T3)
                n84 = Select(t=Scratch_Main_Enum."Close", s=w98, f=w96) -> (s? t:f=w95:T3)
                "Multi Pass Count" <- 0.0 ("Multi Pass Count")
              }
              frame "Start" {
                n85 = Unbundle By Name(w135) -> ("Main Screen.Load En"=w165:refnum<vi>)
                n86 = property class="Bool (strict)"(reference=w165, "Value"=TRUE) -> (reference out=w163:refnum<vi>, error out=w164:errorcluster)  [unwired: 1 in]
                n87 = Close Reference(reference=w163, error in (no error)=w164) -> ()  [unwired: 1 out]
                n88 = local read "Multi Scratch with offset"() -> (w136:bool)
                n89 = case shown="True" w136 {
                  tunnel: w135 -> [_ w168]
                  frame False {
                  }
                  frame True {
                    n90 = local read "Multi Pass Count"() -> (w167:dbl)
                    n91 = Unbundle By Name(w168) -> ("Main Screen.Multi Scratch Pass"=w171:refnum<vi>)
                    n92 = Increment(x=w167) -> (x+1=w166:dbl)
                    n93 = property class="DigNum (strict)"(reference=w171, "Value"=w166) -> (reference out=w169:refnum<vi>, error out=w170:errorcluster)  [unwired: 1 in]
                    n94 = Close Reference(reference=w169, error in (no error)=w170) -> ()  [unwired: 1 out]
                  }
                }
                n95 = Unbundle By Name(w135) -> ("Main Screen.Start Test Temp"=w155:refnum<vi>)
                n96 = Unbundle By Name(w135) -> ("Main Screen.Test Trip"=w143:refnum<vi>)
                n97 = Unbundle By Name(w135) -> ("Main Screen.STOP"=w158:refnum<vi>)
                n98 = property class="Bool (strict)"(reference=w155) -> (reference out=w153:refnum<vi>, error out=w154:errorcluster, "Value"=w156:bool)  [unwired: 1 in]
                n99 = property class="Bool (strict)"(reference=w158) -> (reference out=w160:refnum<vi>, error out=w159:errorcluster, "Value"=w157:bool)  [unwired: 1 in]
                n100 = property class="Bool (strict)"(reference=w143) -> (reference out=w145:refnum<vi>, error out=w144:errorcluster, "Value"=w141:bool)  [unwired: 1 in]
                n101 = Close Reference(reference=w153, error in (no error)=w154) -> ()  [unwired: 1 out]
                n102 = Close Reference(reference=w160, error in (no error)=w159) -> ()  [unwired: 1 out]
                n103 = Equal?(x=w156, y=FALSE) -> (x = y?=w151:bool)
                n104 = Equal?(x=w157, y=TRUE) -> (x = y?=w152:bool)
                n105 = Close Reference(reference=w145, error in (no error)=w144) -> ()  [unwired: 1 out]
                n106 = And(x=w152, y=w151) -> (x .and. y?=w147:bool)
                n107 = Equal?(x=w141, y=TRUE) -> (x = y?=w139:bool)
                n108 = Select(t=Scratch_Main_Enum."Close", s=w147, f=Scratch_Main_Enum."Load") -> (s? t:f=w138:T3)
                n109 = Select(t=Scratch_Main_Enum."Close", s=w139, f=w138) -> (s? t:f=w137:T3)
              }
              frame "Load" {
                n110 = Unbundle By Name(w176) -> ("Main Screen.NL disp 2"=w210:refnum<vi>)
                n111 = Unbundle By Name(w176) -> ("Main Screen.Set Load (N)"=w206:refnum<vi>)
                n112 = property class="DigNum (strict)"(reference=w210) -> (reference out=w208:refnum<vi>, error out=w209:errorcluster, "Value"=w201:dbl)  [unwired: 1 in]
                n113 = property class="DigNum (strict)"(reference=w206) -> (reference out=w205:refnum<vi>, error out=w207:errorcluster, "Value"=w204:dbl)  [unwired: 1 in]
                n114 = Close Reference(reference=w208, error in (no error)=w209) -> ()  [unwired: 1 out]
                n115 = Close Reference(reference=w205, error in (no error)=w207) -> ()  [unwired: 1 out]
                n116 = Subtract(x=w204, y=0.1) -> (x-y=w202:dbl)
                n117 = Greater Or Equal?(x=w201, y=w202) -> (x >= y?=w198:bool)
                n118 = Unbundle By Name(w176) -> ("Main Screen.Start Test Temp"=w190:refnum<vi>)
                n119 = Unbundle By Name(w176) -> ("Main Screen.Test Trip"=w179:refnum<vi>)
                n120 = Unbundle By Name(w176) -> ("Main Screen.STOP"=w193:refnum<vi>)
                n121 = property class="Bool (strict)"(reference=w190) -> (reference out=w188:refnum<vi>, error out=w189:errorcluster, "Value"=w191:bool)  [unwired: 1 in]
                n122 = property class="Bool (strict)"(reference=w193) -> (reference out=w195:refnum<vi>, error out=w194:errorcluster, "Value"=w192:bool)  [unwired: 1 in]
                n123 = property class="Bool (strict)"(reference=w179) -> (reference out=w181:refnum<vi>, error out=w180:errorcluster, "Value"=w177:bool)  [unwired: 1 in]
                n124 = Close Reference(reference=w188, error in (no error)=w189) -> ()  [unwired: 1 out]
                n125 = Close Reference(reference=w195, error in (no error)=w194) -> ()  [unwired: 1 out]
                n126 = Close Reference(reference=w181, error in (no error)=w180) -> ()  [unwired: 1 out]
                n127 = Equal?(x=w191, y=FALSE) -> (x = y?=w186:bool)
                n128 = Equal?(x=w192, y=TRUE) -> (x = y?=w187:bool)
                n129 = Equal?(x=w177, y=TRUE) -> (x = y?=w175:bool)
                n130 = And(x=w187, y=w186) -> (x .and. y?=w183:bool)
                n131 = Select(t=Scratch_Main_Enum."Scratch Forward", s=w198, f=Scratch_Main_Enum."Load") -> (s? t:f=w182:T3)
                n132 = Select(t=Scratch_Main_Enum."Close", s=w183, f=w182) -> (s? t:f=w174:T3)
                n133 = Select(t=Scratch_Main_Enum."Close", s=w175, f=w174) -> (s? t:f=w172:T3)
                "Scratch Forward Temp" <- TRUE ("Scratch Forward Temp")
              }
              frame "Scratch Forward" {
                n134 = flat-sequence {
                  tunnel: w215 -> [w216]
                  tunnel: w214 -> [w222]
                  tunnel: [w221] -> w213
                  tunnel: [w216] -> w212
                  tunnel: w213 -> [_]
                  tunnel: w212 -> [w244]
                  tunnel: [w240] -> w211
                  frame #0 {
                    n135 = local read "Scratch Forward Temp"() -> (w223:bool)
                    n136 = Unbundle By Name(w216) -> ("Main Screen.Scratch Start Test"=w219:refnum<vi>)
                    n137 = case shown="True" w223 {
                      selector: w223 -> [_ w234]
                      tunnel: w216 -> [_ w225]
                      tunnel: w222 -> [w224 w232]
                      tunnel: [w224 w231] -> w221
                      frame False {
                      }
                      frame True {
                        n138 = Unbundle By Name(w225) -> ("Loading.Loading Mode"=w229:refnum<vi>)
                        n139 = property class="Ring (strict)"(reference=w229) -> (reference out=w227:refnum<vi>, error out=w228:errorcluster, "Value"=w226:u16)  [unwired: 1 in]
                        n140 = Not(x=w234) -> (.not. x?=w233:bool)
                        n141 = local write "Scratch Forward Temp"(w233) -> ()
                        n142 = call "Scratch Forward.vi"("error in (no error)"=w232, "main ref"=w225) -> ("error out"=w231:errorcluster, "Distance Moved"=→"Distance Moved":dbl)  [unwired: 8 in]
                        n143 = Close Reference(reference=w227, error in (no error)=w228) -> ()  [unwired: 1 out]
                        n144 = case shown="1" w226 {
                          tunnel: w225 -> [_ w236]
                          frame 0, Default {
                          }
                          frame 1 {
                            n145 = Unbundle By Name(w236) -> ("PID.Ramp"=w237:refnum<vi>)
                            n146 = property class="Bool (strict)"(reference=w237, "Value"=TRUE) -> (reference out=w239:refnum<vi>, error out=w238:errorcluster)  [unwired: 1 in]
                            n147 = Close Reference(reference=w239, error in (no error)=w238) -> ()  [unwired: 1 out]
                          }
                        }
                      }
                    }
                    n148 = property class="Bool (strict)"(reference=w219, "Value"=TRUE) -> (reference out=w220:refnum<vi>, error out=w218:errorcluster)  [unwired: 1 in]
                    n149 = Close Reference(reference=w220, error in (no error)=w218) -> ()  [unwired: 1 out]
                  }
                  frame #1 {
                    n150 = Unbundle By Name(w244) -> ("Motion Module.Motion type:"=w269:refnum<vi>)
                    n151 = Unbundle By Name(w244) -> ("Main Screen.Start Test Temp"=w258:refnum<vi>)
                    n152 = Unbundle By Name(w244) -> ("SWAY.SWAY POSE"=w275:refnum<vi>)
                    n153 = Unbundle By Name(w244) -> ("Main Screen.Test Trip"=w247:refnum<vi>)
                    n154 = Unbundle By Name(w244) -> ("Main Screen.STOP"=w261:refnum<vi>)
                    n155 = property class="DigNum (strict)"(reference=w275) -> (reference out=w274:refnum<vi>, error out=w276:errorcluster, "Value"=w273:sgl)  [unwired: 1 in]
                    n156 = property class="Ring (strict)"(reference=w269) -> (reference out=w270:refnum<vi>, error out=w268:errorcluster, "Value"=w267:u16)  [unwired: 1 in]
                    n157 = local read "Distance Moved"() -> (w272:dbl)
                    n158 = property class="Bool (strict)"(reference=w258) -> (reference out=w256:refnum<vi>, error out=w257:errorcluster, "Value"=w259:bool)  [unwired: 1 in]
                    n159 = property class="Bool (strict)"(reference=w261) -> (reference out=w263:refnum<vi>, error out=w262:errorcluster, "Value"=w260:bool)  [unwired: 1 in]
                    n160 = property class="Bool (strict)"(reference=w247) -> (reference out=w249:refnum<vi>, error out=w248:errorcluster, "Value"=w245:bool)  [unwired: 1 in]
                    n161 = Close Reference(reference=w270, error in (no error)=w268) -> ()  [unwired: 1 out]
                    n162 = Close Reference(reference=w274, error in (no error)=w276) -> ()  [unwired: 1 out]
                    n163 = Close Reference(reference=w256, error in (no error)=w257) -> ()  [unwired: 1 out]
                    n164 = Close Reference(reference=w263, error in (no error)=w262) -> ()  [unwired: 1 out]
                    n165 = Equal?(x=w259, y=FALSE) -> (x = y?=w254:bool)
                    n166 = Close Reference(reference=w249, error in (no error)=w248) -> ()  [unwired: 1 out]
                    n167 = Equal?(x=w260, y=TRUE) -> (x = y?=w255:bool)
                    n168 = Less Or Equal?(x=w273, y=w272) -> (x <= y?=w271:bool)
                    n169 = case shown="0, Default" w267 {
                      tunnel: [Scratch_Main_Enum."Unload" Scratch_Main_Enum."Scratch Backward"] -> w266
                      frame 0, Default {
                        n170 = local write "PID Unload Temp"(TRUE ("PID Unload Temp")) -> ()
                      }
                      frame 1 {
                        "Scratch Backward Temp" <- TRUE
                      }
                    }
                    n171 = And(x=w255, y=w254) -> (x .and. y?=w251:bool)
                    n172 = Equal?(x=w245, y=TRUE) -> (x = y?=w242:bool)
                    n173 = Select(t=w266, s=w271, f=Scratch_Main_Enum."Scratch Forward") -> (s? t:f=w250:T3)
                    n174 = Select(t=Scratch_Main_Enum."Close", s=w251, f=w250) -> (s? t:f=w241:T3)
                    n175 = Select(t=Scratch_Main_Enum."Close", s=w242, f=w241) -> (s? t:f=w240:T3)
                  }
                }
              }
              frame "Scratch Backward" {
                n176 = flat-sequence {
                  tunnel: w285 -> [w287]
                  tunnel: w284 -> [w289]
                  tunnel: [w288] -> w283
                  tunnel: [w287] -> w282
                  tunnel: w283 -> [_]
                  tunnel: w282 -> [w301]
                  tunnel: [w298] -> w281
                  frame #0 {
                    n177 = local read "Scratch Backward Temp"() -> (w286:bool)
                    n178 = case shown="True" w286 {
                      selector: w286 -> [_ w292]
                      tunnel: w287 -> [_ w296]
                      tunnel: w289 -> [w290 w295]
                      tunnel: [w290 w294] -> w288
                      frame False {
                      }
                      frame True {
                        n179 = Not(x=w292) -> (.not. x?=w291:bool)
                        n180 = local write "Scratch Backward Temp"(w291) -> ()
                        n181 = call "Scratch Backward.vi"("error in (no error)"=w295, "main ref"=w296) -> ("error out"=w294:errorcluster, "Distance Moved"=→"Distance Moved Backward":dbl)  [unwired: 8 in]
                      }
                    }
                  }
                  frame #1 {
                    w300 = Scratch_Main_Enum."Close"
                    n182 = Unbundle By Name(w301) -> ("Main Screen.Start Test Temp"=w315:refnum<vi>)
                    n183 = Unbundle By Name(w301) -> ("Main Screen.Test Trip"=w304:refnum<vi>)
                    n184 = Unbundle By Name(w301) -> ("SWAY.SWAY POSE"=w328:refnum<vi>)
                    n185 = Unbundle By Name(w301) -> ("Main Screen.STOP"=w318:refnum<vi>)
                    n186 = property class="DigNum (strict)"(reference=w328) -> (reference out=w327:refnum<vi>, error out=w329:errorcluster, "Value"=w326:sgl)  [unwired: 1 in]
                    n187 = local read "Distance Moved Backward"() -> (w325:dbl)
                    n188 = property class="Bool (strict)"(reference=w315) -> (reference out=w313:refnum<vi>, error out=w314:errorcluster, "Value"=w316:bool)  [unwired: 1 in]
                    n189 = property class="Bool (strict)"(reference=w318) -> (reference out=w320:refnum<vi>, error out=w319:errorcluster, "Value"=w317:bool)  [unwired: 1 in]
                    n190 = property class="Bool (strict)"(reference=w304) -> (reference out=w306:refnum<vi>, error out=w305:errorcluster, "Value"=w302:bool)  [unwired: 1 in]
                    n191 = Close Reference(reference=w327, error in (no error)=w329) -> ()  [unwired: 1 out]
                    n192 = Close Reference(reference=w313, error in (no error)=w314) -> ()  [unwired: 1 out]
                    n193 = Close Reference(reference=w320, error in (no error)=w319) -> ()  [unwired: 1 out]
                    n194 = Close Reference(reference=w306, error in (no error)=w305) -> ()  [unwired: 1 out]
                    n195 = Equal?(x=w316, y=FALSE) -> (x = y?=w311:bool)
                    n196 = Equal?(x=w317, y=TRUE) -> (x = y?=w312:bool)
                    n197 = Greater Or Equal?(x=w326, y=w325) -> (x >= y?=w324:bool)
                    n198 = Equal?(x=w302, y=TRUE) -> (x = y?=w297:bool)
                    n199 = And(x=w312, y=w311) -> (x .and. y?=w308:bool)
                    n200 = Select(t=Scratch_Main_Enum."Unload", s=w324, f=Scratch_Main_Enum."Scratch Backward") -> (s? t:f=w307:T3)
                    n201 = Select(t=w300, s=w308, f=w307) -> (s? t:f=w299:T3)
                    n202 = Select(t=w300, s=w297, f=w299) -> (s? t:f=w298:T3)
                    "PID Unload Temp" <- TRUE ("PID Unload Temp")
                  }
                }
              }
              frame "Unload" {
                n203 = Unbundle By Name(w337) -> ("Main Screen.Load En"=w345:refnum<vi>)
                n204 = local read "Multi Scratch with offset"() -> (w330:bool)
                n205 = property class="Bool (strict)"(reference=w345, error in=w343, "Value"=FALSE) -> (reference out=w347:refnum<vi>, error out=w346:errorcluster)
                n206 = Close Reference(reference=w347, error in (no error)=w346) -> (error out=w344:errorcluster)
                n207 = case shown="False" w330 {
                  tunnel: w337 -> [w380 _]
                  frame False {
                    n208 = Unbundle By Name(w380) -> ("Main Screen.Scratch Start Test"=w383:refnum<vi>)
                    n209 = property class="Bool (strict)"(reference=w383, "Value"=FALSE) -> (reference out=w384:refnum<vi>, error out=w382:errorcluster)  [unwired: 1 in]
                    n210 = Close Reference(reference=w384, error in (no error)=w382) -> ()  [unwired: 1 out]
                  }
                  frame True {
                  }
                }
                n211 = disable-structure shown="Disabled" {
                  disable-tunnel: w344 -> [w387 w388]
                  disable-tunnel: [w386 w388] -> w350
                  disable-tunnel: w337 -> [w385 _]
                  frame Disabled {
                    n212 = call "Test Stop.vi"("error in (no error)"=w387, "Data Cluster"=w385) -> ("error out"=w386:errorcluster)  [unwired: 9 in]
                  }
                  frame Enabled {
                  }
                }
                n213 = call "Stall Data Flow.vim"("value in"=w350, "milliseconds to wait"=u32 400) -> ("value out"=w342:errorcluster)  [unwired: 1 out]
                n214 = call "Sway Stop.vi"("error in (no error)"=w342, "main ref"=w337) -> ("error out"=w356:errorcluster)  [unwired: 9 in]
                n215 = call "PID stop.vi"("error in (no error)"=w356, "main ref"=w337) -> ("error out"=w357:errorcluster)  [unwired: 9 in]
                n216 = call "Stall Data Flow.vim"("value in"=w357, "milliseconds to wait"=u32 400) -> ("value out"=w353:errorcluster)  [unwired: 1 out]
                n217 = call "PID UNLOAD.vi"("error in (no error)"=w353, "main ref"=w337) -> ("error out"=w352:errorcluster)  [unwired: 9 in]
                n218 = call "HEAVE WRITE FGV.vi"("Enum - Menu"=Heave_Write_enum."WRITE", "error in (no error)"=w352, "main ref"=w337) -> ("error out"=w355:errorcluster)  [unwired: 8 in]
                n219 = call "SWAY UNIFORM SPEED STOP.vi"("error in (no error)"=w355, "Data Cluster"=w337) -> ("error out"=w349:errorcluster)  [unwired: 9 in]
                n220 = Unbundle By Name(w337) -> ("Main Screen.Test Trip"=w338:refnum<vi>)
                n221 = Unbundle By Name(w337) -> ("Main Screen.Start Test Temp"=w368:refnum<vi>)
                n222 = Unbundle By Name(w337) -> ("Main Screen.STOP"=w371:refnum<vi>)
                n223 = Unbundle By Name(w337) -> ("Motion Module.Motion type:"=w378:refnum<vi>)
                n224 = property class="Bool (strict)"(reference=w338) -> (reference out=w340:refnum<vi>, error out=w339:errorcluster, "Value"=w335:bool)  [unwired: 1 in]
                n225 = property class="Bool (strict)"(reference=w368) -> (reference out=w366:refnum<vi>, error out=w367:errorcluster, "Value"=w369:bool)  [unwired: 1 in]
                n226 = property class="Bool (strict)"(reference=w371) -> (reference out=w373:refnum<vi>, error out=w372:errorcluster, "Value"=w370:bool)  [unwired: 1 in]
                n227 = property class="Ring (strict)"(reference=w378) -> (reference out=w379:refnum<vi>, error out=w377:errorcluster, "Value"=w376:u16)  [unwired: 1 in]
                n228 = Close Reference(reference=w340, error in (no error)=w339) -> ()  [unwired: 1 out]
                n229 = call "Stall Data Flow.vim"("value in"=w349, "milliseconds to wait"=u32 500) -> ("value out"=w359:errorcluster)  [unwired: 1 out]
                n230 = Close Reference(reference=w366, error in (no error)=w367) -> ()  [unwired: 1 out]
                n231 = Close Reference(reference=w373, error in (no error)=w372) -> ()  [unwired: 1 out]
                n232 = Equal?(x=w335, y=TRUE) -> (x = y?=w332:bool)
                n233 = Equal?(x=w369, y=FALSE) -> (x = y?=w364:bool)
                n234 = Close Reference(reference=w379, error in (no error)=w377) -> ()  [unwired: 1 out]
                n235 = Equal?(x=w370, y=TRUE) -> (x = y?=w365:bool)
                n236 = And(x=w365, y=w364) -> (x .and. y?=w361:bool)
                n237 = case shown="1" w376 {
                  tunnel: w359 -> [w392 w393]
                  tunnel: w337 -> [w391 _]
                  tunnel: [w390 w393] -> w375
                  frame 0, Default {
                    n238 = call "Scratch Backward for forward.vi"("error in (no error)"=w392, "main ref"=w391) -> ("error out"=w390:errorcluster, "Distance Moved"=→"Distance Moved unload":dbl)  [unwired: 8 in]
                  }
                  frame 1 {
                  }
                }
                n239 = Select(t=Scratch_Main_Enum."Close", s=w361, f=Scratch_Main_Enum."Offest") -> (s? t:f=w334:T3)
                n240 = Select(t=Scratch_Main_Enum."Close", s=w332, f=w334) -> (s? t:f=w331:T3)
              }
              frame "Offest" {
                n241 = Unbundle By Name(w398) -> ("Motion Module.Motion type:"=w429:refnum<vi>)
                n242 = local read "Multi Pass Count"() -> (w396:dbl)
                n243 = property class="Ring (strict)"(reference=w429) -> (reference out=w430:refnum<vi>, error out=w428:errorcluster, "Value"=w427:u16)  [unwired: 1 in]
                n244 = local read "Multi Scratch with offset"() -> (w397:bool)
                n245 = Unbundle By Name(w398) -> ("Motion Module.No of Scratch"=w400:refnum<vi>)
                n246 = Close Reference(reference=w430, error in (no error)=w428) -> ()  [unwired: 1 out]
                n247 = property class="DigNum (strict)"(reference=w400) -> (reference out=w401:refnum<vi>, error out=w399:errorcluster, "Value"=w395:dbl)  [unwired: 1 in]
                n248 = Greater Or Equal?(x=w396, y=w395) -> (x >= y?=w394:bool)
                n249 = case shown="True" w397 {
                  tunnel: w398 -> [w432 w437]
                  tunnel: w394 -> [_ w438]
                  frame False {
                    n250 = Unbundle By Name(w432) -> ("Main Screen.Scratch Start Test"=w435:refnum<vi>)
                    n251 = property class="Bool (strict)"(reference=w435, "Value"=FALSE) -> (reference out=w436:refnum<vi>, error out=w434:errorcluster)  [unwired: 1 in]
                    n252 = Close Reference(reference=w436, error in (no error)=w434) -> ()  [unwired: 1 out]
                  }
                  frame True {
                    n253 = case shown="True" w438 {
                      tunnel: w437 -> [_ w439]
                      frame False {
                      }
                      frame True {
                        n254 = Unbundle By Name(w439) -> ("Main Screen.Scratch Start Test"=w442:refnum<vi>)
                        n255 = property class="Bool (strict)"(reference=w442, "Value"=FALSE) -> (reference out=w443:refnum<vi>, error out=w441:errorcluster)  [unwired: 1 in]
                        n256 = Close Reference(reference=w443, error in (no error)=w441) -> ()  [unwired: 1 out]
                      }
                    }
                  }
                }
                n257 = case shown="0, Default" w427 {
                  tunnel: w398 -> [w447 w476]
                  tunnel: w431 -> [w450 w475]
                  tunnel: [w445 w474] -> w426
                  tunnel: [w448 Scratch_Main_Enum."Close"] -> w411
                  tunnel: w395 -> [w444 _]
                  frame 0, Default {
                    n258 = Unbundle By Name(w447) -> ("SWAY.SWAY POSE"=w452:refnum<vi>)
                    n259 = local read "Distance Moved unload"() -> (w455:dbl)
                    n260 = property class="DigNum (strict)"(reference=w452, error in=w450) -> (reference out=w453:refnum<vi>, error out=w451:errorcluster, "Value"=w454:sgl)
                    n261 = Greater Or Equal?(x=w454, y=w455) -> (x >= y?=w449:bool)
                    n262 = Close Reference(reference=w453, error in (no error)=w451) -> (error out=w446:errorcluster)
                    n263 = case shown="True" w449 {
                      tunnel: [Scratch_Main_Enum."Offest" w461] -> w448
                      tunnel: w447 -> [_ w464]
                      tunnel: w446 -> [w456 w463]
                      tunnel: [w456 w462] -> w445
                      tunnel: w444 -> [_ w458]
                      frame False {
                      }
                      frame True {
                        n264 = local read "Multi Scratch with offset"() -> (w460:bool)
                        n265 = call "Surge Forward in Scratch.vi"("error in (no error)"=w463, "main ref"=w464) -> ("error out"=w462:errorcluster)  [unwired: 9 in]
                        n266 = local read "Multi Pass Count"() -> (w459:dbl)
                        n267 = case shown="True" w460 {
                          tunnel: [Scratch_Main_Enum."Close" w470] -> w461
                          tunnel: w459 -> [_ w467]
                          tunnel: w458 -> [_ w466]
                          frame False {
                          }
                          frame True {
                            n268 = Increment(x=w467) -> (x+1=w469:dbl)
                            n269 = Greater Or Equal?(x=w467, y=w466) -> (x >= y?=w468:bool)
                            n270 = local write "Multi Pass Count"(w469) -> ()
                            n271 = case shown="True" w468 {
                              tunnel: [Scratch_Main_Enum."Start" Scratch_Main_Enum."Close"] -> w470
                              frame False {
                              }
                              frame True {
                              }
                            }
                          }
                        }
                      }
                    }
                  }
                  frame 1 {
                    n272 = call "Surge Forward in Scratch.vi"("error in (no error)"=w475, "main ref"=w476) -> ("error out"=w474:errorcluster)  [unwired: 9 in]
                  }
                }
                n273 = Close Reference(reference=w401, error in (no error)=w399) -> ()  [unwired: 1 out]
                n274 = Unbundle By Name(w398) -> ("Main Screen.Start Test Temp"=w419:refnum<vi>)
                n275 = Unbundle By Name(w398) -> ("Main Screen.Test Trip"=w407:refnum<vi>)
                n276 = Unbundle By Name(w398) -> ("Main Screen.STOP"=w422:refnum<vi>)
                n277 = property class="Bool (strict)"(reference=w419) -> (reference out=w417:refnum<vi>, error out=w418:errorcluster, "Value"=w420:bool)  [unwired: 1 in]
                n278 = property class="Bool (strict)"(reference=w422) -> (reference out=w424:refnum<vi>, error out=w423:errorcluster, "Value"=w421:bool)  [unwired: 1 in]
                n279 = property class="Bool (strict)"(reference=w407) -> (reference out=w409:refnum<vi>, error out=w408:errorcluster, "Value"=w405:bool)  [unwired: 1 in]
                n280 = Close Reference(reference=w417, error in (no error)=w418) -> ()  [unwired: 1 out]
                n281 = Close Reference(reference=w424, error in (no error)=w423) -> ()  [unwired: 1 out]
                n282 = Close Reference(reference=w409, error in (no error)=w408) -> ()  [unwired: 1 out]
                n283 = Equal?(x=w420, y=FALSE) -> (x = y?=w415:bool)
                n284 = Equal?(x=w421, y=TRUE) -> (x = y?=w416:bool)
                n285 = Equal?(x=w405, y=TRUE) -> (x = y?=w404:bool)
                n286 = And(x=w416, y=w415) -> (x .and. y?=w412:bool)
                n287 = Select(t=Scratch_Main_Enum."Close", s=w412, f=w411) -> (s? t:f=w403:T3)
                n288 = Select(t=Scratch_Main_Enum."Close", s=w404, f=w403) -> (s? t:f=w402:T3)
              }
              frame "Close" {
                n289 = Unbundle By Name(w479) -> ("Main Screen.Test Trip"=w482:refnum<vi>)
                n290 = property class="Bool (strict)"(reference=w482) -> (reference out=w484:refnum<vi>, error out=w483:errorcluster, "Value"=w480:bool)  [unwired: 1 in]
                n291 = Close Reference(reference=w484, error in (no error)=w483) -> ()  [unwired: 1 out]
                n292 = Equal?(x=w480, y=TRUE) -> (x = y?=w478:bool)
                n293 = local write "Multi Scratch with offset"(FALSE ("Multi Scratch with offset")) -> ()
                n294 = case shown="True" w478 {
                  tunnel: w487 -> [w491 w492]
                  tunnel: [w490 w492] -> w485
                  tunnel: w479 -> [w489 _]
                  frame False {
                    n295 = call "Sway Stop.vi"("error in (no error)"=w491, "main ref"=w489) -> ("error out"=w490:errorcluster)  [unwired: 9 in]
                  }
                  frame True {
                  }
                }
                n296 = case shown="False" w478 {
                  tunnel: w479 -> [w493 _]
                  frame False {
                    n297 = Unbundle By Name(w493) -> ("Loading.Loading Mode"=w501:refnum<vi>)
                    n298 = Unbundle By Name(w493) -> ("Main Screen.Start Test"=w515:refnum<vi>)
                    n299 = Unbundle By Name(w493) -> ("Main Screen.STOP"=w504:refnum<vi>)
                    n300 = Unbundle By Name(w493) -> ("Main Screen.Start Test Temp"=w505:refnum<vi>)
                    n301 = Unbundle By Name(w493) -> ("Main Screen.Load En"=w513:refnum<vi>)
                    n302 = property class="Ring (strict)"(reference=w501) -> (reference out=w499:refnum<vi>, error out=w500:errorcluster, "Value"=w498:u16)  [unwired: 1 in]
                    n303 = Close Reference(reference=w499, error in (no error)=w500) -> ()  [unwired: 1 out]
                    n304 = property class="Bool (strict)"(reference=w504, "Value"=FALSE, "Visible"=TRUE) -> (reference out=w502:refnum<vi>, error out=w503:errorcluster)  [unwired: 1 in]
                    n305 = property class="Bool (strict)"(reference=w505, "Value"=FALSE) -> (reference out=w507:refnum<vi>, error out=w506:errorcluster)  [unwired: 1 in]
                    n306 = property class="Bool (strict)"(reference=w513, "Value"=FALSE) -> (reference out=w511:refnum<vi>, error out=w512:errorcluster)  [unwired: 1 in]
                    n307 = property class="Bool (strict)"(reference=w515, "Value"=FALSE, "Visible"=TRUE) -> (reference out=w517:refnum<vi>, error out=w516:errorcluster)  [unwired: 1 in]
                    n308 = case shown="1" w498 {
                      tunnel: w493 -> [_ w521]
                      frame 0, Default {
                      }
                      frame 1 {
                        n309 = Unbundle By Name(w521) -> ("PID.Ramp"=w522:refnum<vi>)
                        n310 = property class="Bool (strict)"(reference=w522, "Value"=FALSE) -> (reference out=w524:refnum<vi>, error out=w523:errorcluster)  [unwired: 1 in]
                        n311 = Close Reference(reference=w524, error in (no error)=w523) -> ()  [unwired: 1 out]
                      }
                    }
                    n312 = Close Reference(reference=w502, error in (no error)=w503) -> ()  [unwired: 1 out]
                    n313 = Close Reference(reference=w507, error in (no error)=w506) -> ()  [unwired: 1 out]
                    n314 = Close Reference(reference=w511, error in (no error)=w512) -> ()  [unwired: 1 out]
                    n315 = Close Reference(reference=w517, error in (no error)=w516) -> ()  [unwired: 1 out]
                    n316 = Unbundle By Name(w493) -> ("Main Screen.Scratch Start Test"=w496:refnum<vi>)
                    n317 = property class="Bool (strict)"(reference=w496, "Value"=FALSE) -> (reference out=w497:refnum<vi>, error out=w495:errorcluster)  [unwired: 1 in]
                    n318 = Close Reference(reference=w497, error in (no error)=w495) -> ()  [unwired: 1 out]
                  }
                  frame True {
                  }
                }
              }
            }
            n319 = Wait (ms)(milliseconds to wait=u32 200) -> ()  [unwired: 1 out]
          }
        }
      }
    }
    frame Error {
    }
  }
